vi "Main_Andor_Multi_ver2.vi"() -> ()   [LabVIEW 2014]
doc: "This is the main user interface of the Raman spectroscopy system."
uses:
  C:/Users/light/Desktop/Chuanzhen/Labview/Raman/dll/Thorlabs.MotionControl.Controls.dll
  dll/Thorlabs.MotionControl.Controls.dll
  <userlib>/atmcd64d.llb/AcquisitionMode_mode typedef.ctl
  <userlib>/atmcd64d.llb/ReadMode_mode typedef.ctl
  <userlib>/atmcd64d.llb/Shutter_mode typedef.ctl
  <userlib>/atmcd64d.llb/Shutter_type typedef.ctl
  <userlib>/atmcd64d.llb/TriggerMode_mode typedef.ctl
  TypeDef/GalvoInput.ctl
  <userlib>/atmcd64d.llb/Error Code Enum typedef.ctl
  TypeDef/States.ctl
  TypeDef/StageDeviceOut.ctl
  TypeDef/StageHandleIn.ctl
  <vilib>/Utility/miscctls.llb/LVPoint32TypeDef.ctl
  TypeDef/LaserSpot.ctl
  C:/Users/light/Desktop/Chuanzhen/Labview/Raman/dll/ThorLabs.MotionControl.KCube.DCServoCLI.dll
  dll/ThorLabs.MotionControl.KCube.DCServoCLI.dll
  TypeDef/StageSelect.ctl
  TypeDef/inputImages.ctl
  C:/Users/light/Desktop/Chuanzhen/Labview/Raman/dll/Thorlabs.MotionControl.GenericMotorCLI.dll
  dll/Thorlabs.MotionControl.GenericMotorCLI.dll
panel:
  out "Boolean":bool
  in  "Tab Control":enum32{"Main", "Andor", "Galvo"}(tab)
  in  "Scan Range":T1={"Ver_V/H"=0.35, "Hor_V/W"=0.35, "Ver_r"=5.0, "Hor_r"=5.0}
  in  "Scan Resolusion":T2={"Ver_V"=0.35, "Hor_H"=0.35, "Ver_Pix"=214.0, "Hor_Pix"=200.0}
  in  "Galvo Center":bool
  out "Galvo":bool
  out "Spot Y":dbl
  out "Spot X":dbl
  in  "Box":cluster{"Width":dbl, " Height":dbl}={"Width"=200.0, " Height"=214.0}
  in  "Quit":bool
  out "Height":i32=480
  out "Width":i32=640
  out "FPS":dbl=6.258409738085552
  in  "Blacklevel Offset":i32(slide) min=0 max=255 scale=0.0..255.0
  in  "Frame rate":dbl(slide)=9.996754624578479 min=0.5 max=17.288905497022668 step=5.487719298245614e-05 scale=0.5..17.288905497022668 scale format="%^#_3g"
  in  "Pixel clock":i32(slide)=20 min=7 max=86 scale=7.0..86.0
  in  "Exposure time (ms)":dbl(slide)=11.094175438596492 min=0.008982456140350877 max=99.9862456140351 step=0.05487719298245614 scale=0.008982456140350877..99.9862456140351 scale format="%#.3g"
  in  "Edge Filter Enable / Disable":bool
  in  "Edge Filter":i32(ring)=2 items=["High"=1, "Low"=2]
  in  "Blacklevel compensation":bool
  in  "Hotpixel correction 2":bool
  in  "Master Gain":i32(slide) min=0 max=100 scale=0.0..100.0
  in  "Autogain":bool
  out "Bits/Pixel":i32=8
  in  "Camera ID":u32
  out "Live video":picture caption="600 x 480"
  in  "Focus":bool
  out "ZoomRatio":dbl format="%#_2g"
  in  "Jog size (um)":dbl=2.0
  out "Delay (s)":dbl=0.9 format="%#_13g"
  out "Focal plane (mm)":dbl
  out "Initialization finished":bool
  in  "Aim":bool
  in  "Pixel Size X (um)":dbl=0.0877
  in  "LaserSpot":bool
  in  "Pixel Size Y (um)":dbl=0.0877
  in  "ImageSnap":bool
  in  "Left":bool
  in  "Right":bool
  in  "Up":bool
  in  "Down":bool
  in  "X axis_R":bool
  in  "X axis_L":bool
  in  "Reset":bool
  out "Z_axis":dbl
  out "X_axis":dbl
  out "Y_axis":dbl
  in  "Y axis_B":bool
  in  "Y axis_F":bool
  in  "Z axis_u":bool
  in  "Z axis_d":bool
  in  "Jogstep of Z axis":T3(radio)=enum."10step"
  in  "MoveTo":bool
  in  "Velocity: X and Y axis":T4(radio)=enum."0.05mm"
  in  "Scan":bool
  in  "Save Path":path=path "C:/Users/light/Desktop/Chuanzhen/test"
  in  "Destination":dbl=12.0
  out "Frame_X":dbl
  out "Frame_Y":dbl
  out "Total_Frame_X":dbl
  out "Total_Frame_Y":dbl
  in  "Galvo Stop":bool
  in  "Galvo Scan":bool
  out "Andor":bool
  out "CurrentFrame":i32
  in  "Set":bool
  in  "AndorSnap":bool
  out "SaveStatus":bool
  in  "FilePath":string="C:\\Users\\light\\Desktop\\Chuanzhen\\Image\\ImageReconstruct\\data\\TempSpectralData"
  in  "Exit":bool
  out "ShutDown":cluster{"CoolOff":bool, "ShutDown":bool}
  in  "Mode":T10={"AcqMode"=enum."Single Scan", "ReadMode"=enum."Single-Track", "ShutterMode"=enum."Auto", "GateMode"=enum."TTL High", "TriggerMode"=enum."Internal"}
  in  "AcqSet":T11={"openingtime"=0, "closingtime/ms"=0, "ExposureTime/s"=0.1, "AccumCycTime"=0.0, "AccumCycNum"=1, "KineticNum"=1, "KineticTime"=0.0} {"KineticTime" format="%.5f"; "AccumCycNum" format="%.5f"; "AccumCycTime" format="%.5f"; "ExposureTime/s" format="%.5f"; "closingtime/ms" format="%.2f"; "openingtime" format="%.2f"}
  out "Timing":T12 {"kinetic" format="%.7f"; "accumulate" format="%.7f"; "exposure" format="%.7f"}
  out "SetOut":T13
  in  "MultiTrack":cluster{"StartRow":i32, "EndRow":i32}={"StartRow"=131, "EndRow"=143}
  out "SetStatus":bool
  out "CurrentTemp":i32
  out "DevInit":bool
  out "DevSize":cluster{"xpixels":i32, "ypixels":i32}
  out "HardWVersion":T14
  out "SoftWVersion":T15
  out "Speeds":T16
  in  "TargetTemp":i32=-50
  out "CoolerON":T17
  out "GetStatus":T18
  in  "YOffset":dbl=8.2 caption="Offset"
  in  "XOffset":dbl=4.0 caption="Offset"
  out "Sample Rate":dbl=1000.0 format="%0.2f"
  out "Waveform Graph":waveform(dbl)[](graph)=[{"t0"=timestamp(0 s since 1904-01-01), "dt"=0.001, "Y"=[]}]
  in  "ZOffset":dbl caption="Offset"
  in  "Galvo":T19={"Sample Rate"=1000.0, "Sample Clock Source"="OnboardClock", "Max Voltage"=10.0, "Min Voltage"=-10.0, "Physical Channel(s)"="Dev1/ao0,Dev1/ao1,Dev1/ao3"}
  in  "Stage Control":enum32{"X axis", "Y axis", "Z axis"}(tab)
  in  "X axis":refnum<k24>(container)
  in  "Y axis":refnum<k24>(container)
  in  "Z axis":refnum<k24>(container)
  # "Camera Control"
  # "Objective: CFI Plan Fluor ELWD 60x (1.27 NA) \nThe depth of field: 1.78 um\nPixel Size: 0.0877um/px"
  # "Attention: \ndon't click button very fast"
  # "Motor Control"
  # "Aim"
  # "Auto Focus"
  # "Adjust laser spot lightly"
  # "Stage Scan"
  # "Total_Frame"
  # "Current_Frame"
  # "X"
  # "Y"
  # "Focus distance ia about 2mm"
  # "Jogstep:"
  # "0.00003mm/step"
  # "Stepsize:"
  # "Kinetics->SignleTrack"
  # "Galvo Control"
  # "50Hz->1s"
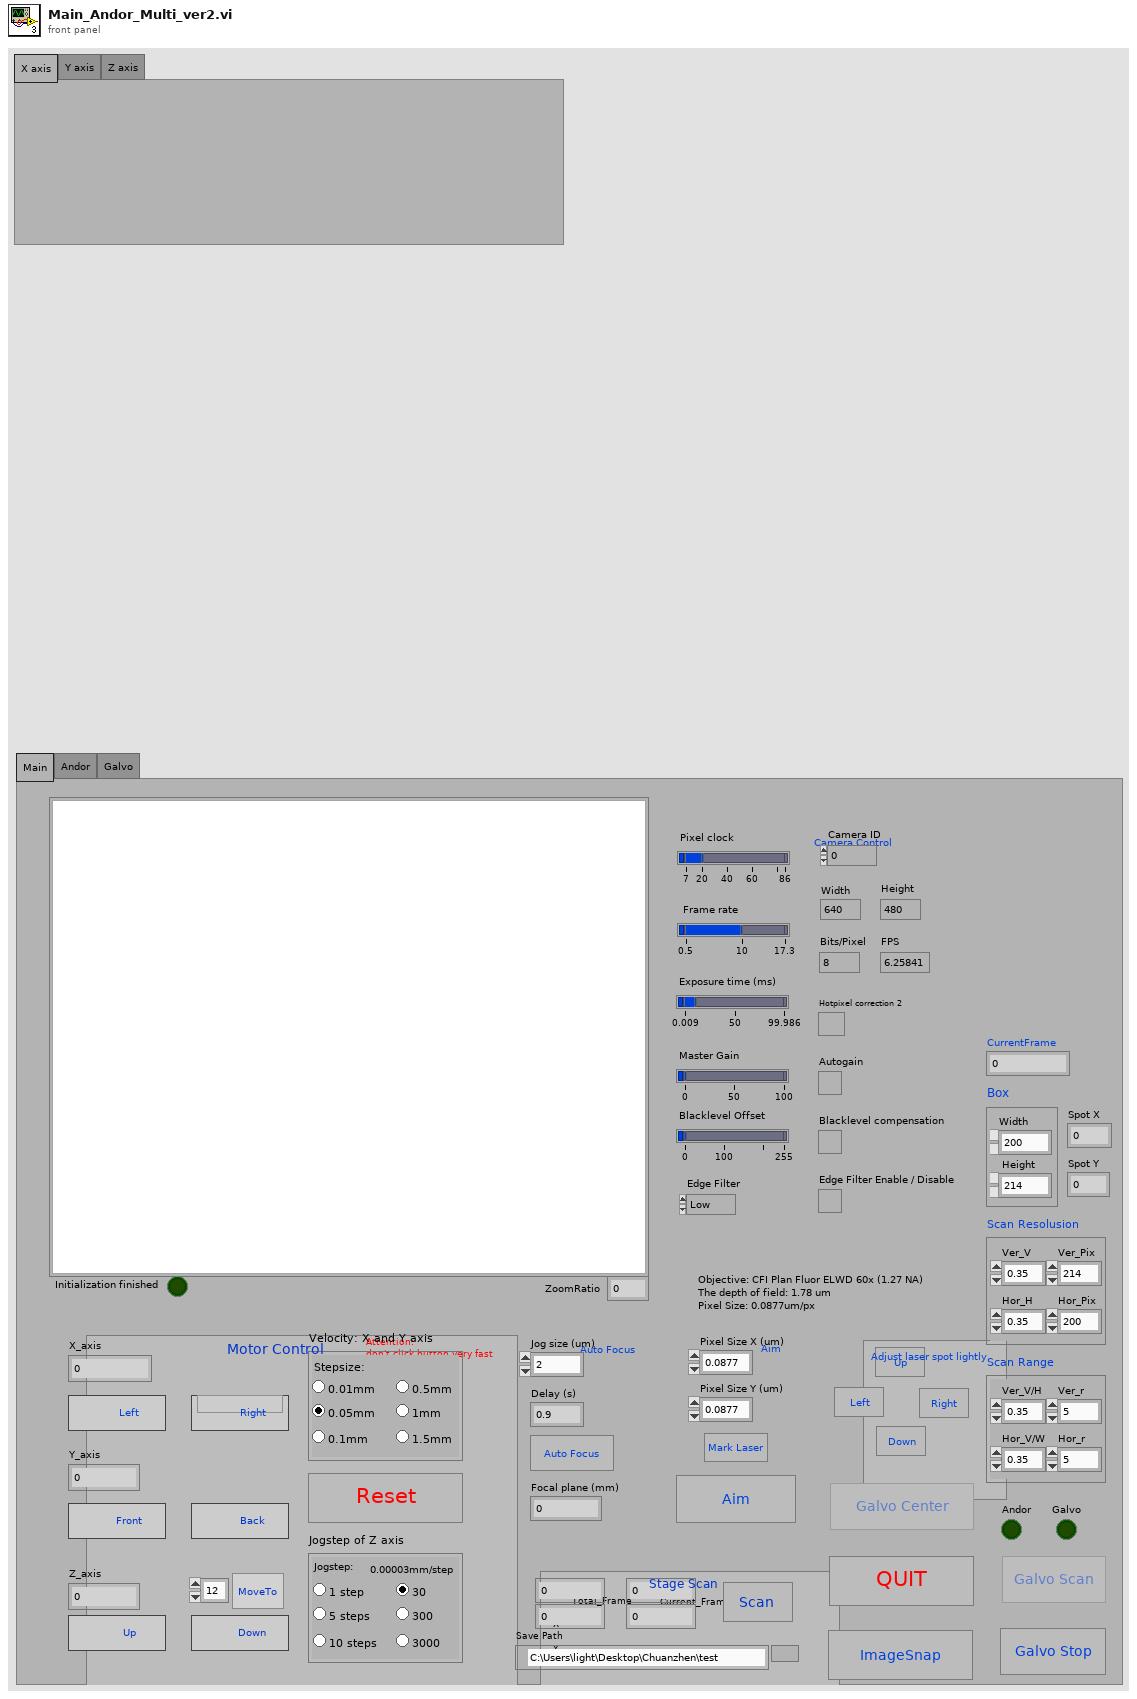
[diagram p1: front panel]
types:
  T1 = cluster{"Ver_V/H":dbl, "Hor_V/W":dbl, "Ver_r":dbl, "Hor_r":dbl}
  T2 = cluster{"Ver_V":dbl, "Hor_H":dbl, "Ver_Pix":dbl, "Hor_Pix":dbl}
  T3 = enum32{"1step", "2step", "5step", "10step", "15step", "20step"}
  T4 = enum32{"0.01mm", "0.05mm", "0.1mm", "0.5mm", "1mm", "1.5mm"}
  T5 = typedef "AcquisitionMode_mode typedef.ctl" = enum16{"Reserved (0)", "Single Scan", "Accumulate", "Kinetics", "Fast Kinetics", "Run Till Abort", "Reserved (6)", "Reserved (7)", "Reserved (8)", "Time Delayed Integration"}
  T6 = typedef "ReadMode_mode typedef.ctl" = enum16{"Full Vertical Binning", "Multi-Track", "Random-Track", "Single-Track", "Image"}
  T7 = typedef "Shutter_mode typedef.ctl" = enum16{"Auto", "Open", "Close", "N/A (3)", "Open FVB Series", "Open Any Series"}
  T8 = typedef "Shutter_type typedef.ctl" = enum16{"TTL Low", "TTL High"}
  T9 = typedef "TriggerMode_mode typedef.ctl" = enum16{"Internal", "External", "N/A (2)", "N/A (3)", "N/A (4)", "N/A (5)", "External Start", "External Exposure (Bulb)", "N/A (8)", "External FVB EM", "Software", "N/A (11)", "External Charge Shifting"}
  T10 = cluster{"AcqMode":T5, "ReadMode":T6, "ShutterMode":T7, "GateMode":T8, "TriggerMode":T9}
  T11 = cluster{"openingtime":i32, "closingtime/ms":i32, "ExposureTime/s":sgl, "AccumCycTime":sgl, "AccumCycNum":i32, "KineticNum":i32, "KineticTime":sgl}
  T12 = cluster{"exposure":sgl, "accumulate":sgl, "kinetic":sgl}
  T13 = cluster{"Height":i32, "Width":i32, "bottom":i32, "gap":i32}
  T14 = cluster{"PCB":u32, "Flex":u32, "dummy1":u32, "dummy2":u32, "dummy3":u32, "dummy4":u32}
  T15 = cluster{"eprom":u32, "cofFile":u32, "vxdRev":u32, "vxdVer":u32, "dllRev":u32, "dllVer":u32}
  T16 = cluster{"NVS":i32, "VS":i32, "NHS":dbl, "HS":i32}
  T17 = cluster{"SetTemp":bool, "CoolerOn":bool, "Stablized":bool}
  T18 = cluster{"GetDetector":bool, "GetHardVer":bool, "GetNVS":bool, "GetVS":bool, "GetSotfVer":bool, "GetNHS":bool, "GetHS":bool}
  T19 = typedef "GalvoInput.ctl" = cluster{"Sample Rate":dbl, "Sample Clock Source":tag, "Max Voltage":dbl, "Min Voltage":dbl, "Physical Channel(s)":tag}
  T20 = typedef "LaserSpot.ctl" = cluster{"Laser X":dbl, "Laser Y":dbl}
  T21 = cluster{"left":i16, "top":i16, "right":i16, "bottom":i16}
  T22 = typedef "LVPoint32TypeDef.ctl" = cluster{"Horizontal":i32, "Vertical":i32}
  T23 = typedef "StageHandleIn.ctl" = cluster{"Z StageHandle in":refnum<k24>, "X StageHandle in":refnum<k24>, "Y StageHandle in":refnum<k24>}
  T24 = typedef "StageDeviceOut.ctl" = cluster{"Device Z":refnum<k24>, "Device X":refnum<k24>, "Device Y":refnum<k24>}
  T25 = typedef "States.ctl" = enum16{"Initialize", "CMOS live", "Shut down"}
  T26 = enum8{"Enabled", "Disabled", "Disabled and Grayed Out"}
  T27 = cluster{"Width":u16, "Style":enum32{"Solid", "Dash", "Dot", "DashDot", "DashDotDot"}}
  T28 = typedef "StageSelect.ctl" = enum16{"X axis", "Y axis", "Z axis"}
  T29 = typedef "inputImages.ctl" = cluster{"Image2":u8[][], "Image3":u8[][], "Image4":u8[][], "Image1":u8[][]}
  T30 = typedef "Error Code Enum typedef.ctl" = enum32{"N/A (0)", "DRV_ERROR_CODES", "DRV_SUCCESS", "DRV_VXDNOTINSTALLED", "DRV_ERROR_SCAN", "DRV_ERROR_CHECK_SUM", "DRV_ERROR_FILELOAD", "DRV_UNKNOWN_FUNC", "DRV_ERROR_VXD_INIT", "DRV_ERROR_ADDRESS", "DRV_ERROR_PAGELOCK", "DRV_ERROR_PAGEUNLOCK", "DRV_ERROR_BOARDTEST", "DRV_ERROR_ACK", "DRV_ERROR_UP_FIFO", "DRV_ERROR_PATTERN", "N/A (16)", "DRV_ACQUISITION_ERRORS", "DRV_ACQ_BUFFER", "DRV_ACQ_DOWNFIFO_FULL", "DRV_PROC_UNKONWN_INSTRUCTION", "DRV_ILLEGAL_OP_CODE", "DRV_KINETIC_TIME_NOT_MET", "DRV_ACCUM_TIME_NOT_MET", "DRV_NO_NEW_DATA", "N/A (25)", "DRV_SPOOLERROR", "N/A (27)", "N/A (28)", "N/A (29)", "N/A (30)", "N/A (31)", "N/A (32)", "DRV_TEMPERATURE_CODES", "DRV_TEMPERATURE_OFF", "DRV_TEMPERATURE_NOT_STABILIZED", "DRV_TEMPERATURE_STABILIZED", "DRV_TEMPERATURE_NOT_REACHED", "DRV_TEMPERATURE_OUT_RANGE", "DRV_TEMPERATURE_NOT_SUPPORTED", "DRV_TEMPERATURE_DRIFT", "N/A (41)", "N/A (42)", "N/A (43)", "N/A (44)", "N/A (45)", "N/A (46)", "N/A (47)", "N/A (48)", "DRV_GENERAL_ERRORS", "DRV_INVALID_AUX", "DRV_COF_NOTLOADED", "DRV_FPGAPROG", "DRV_FLEXERROR", "DRV_GPIBERROR", "N/A (55)", "N/A (56)", "N/A (57)", "N/A (58)", "N/A (59)", "N/A (60)", "N/A (61)", "N/A (62)", "N/A (63)", "DRV_DATATYPE", "DRV_DRIVER_ERRORS", "DRV_P1INVALID", "DRV_P2INVALID", "DRV_P3INVALID", "DRV_P4INVALID", "DRV_INIERROR", "DRV_COFERROR", "DRV_ACQUIRING", "DRV_IDLE", "DRV_TEMPCYCLE", "DRV_NOT_INITIALIZED", "DRV_P5INVALID", "DRV_P6INVALID", "DRV_INVALID_MODE", "DRV_INVALID_FILTER", "DRV_I2CERRORS", "DRV_I2CDEVNOTFOUND", "DRV_I2CTIMEOUT", "DRV_P7INVALID", "N/A (84)", "N/A (85)", "N/A (86)", "N/A (87)", "N/A (88)", "N/A (89)", "DRV_IOCERROR", "DRV_VRMVERSIONERROR"}
  T31 = typedef "StageHandleOut.ctl" = cluster{"Z StageHandle out":refnum<k24>, "X StageHandle out":refnum<k24>, "Y StageHandle out":refnum<k24>}
  T32 = typedef "LVBoundsTypeDef.ctl" = cluster{"Width":u32, "Height":u32}
  T33 = typedef "imagedata.ctl" = cluster{"image type":i32, "image depth":i32, "image":u8[], "mask":u8[], "colors":u32[], "Rectangle":cluster{"left":i16, "top":i16, "right":i16, "bottom":i16}}
  T34 = typedef "LVPositionTypeDef.ctl" = cluster{"Left":i32, "Top":i32}
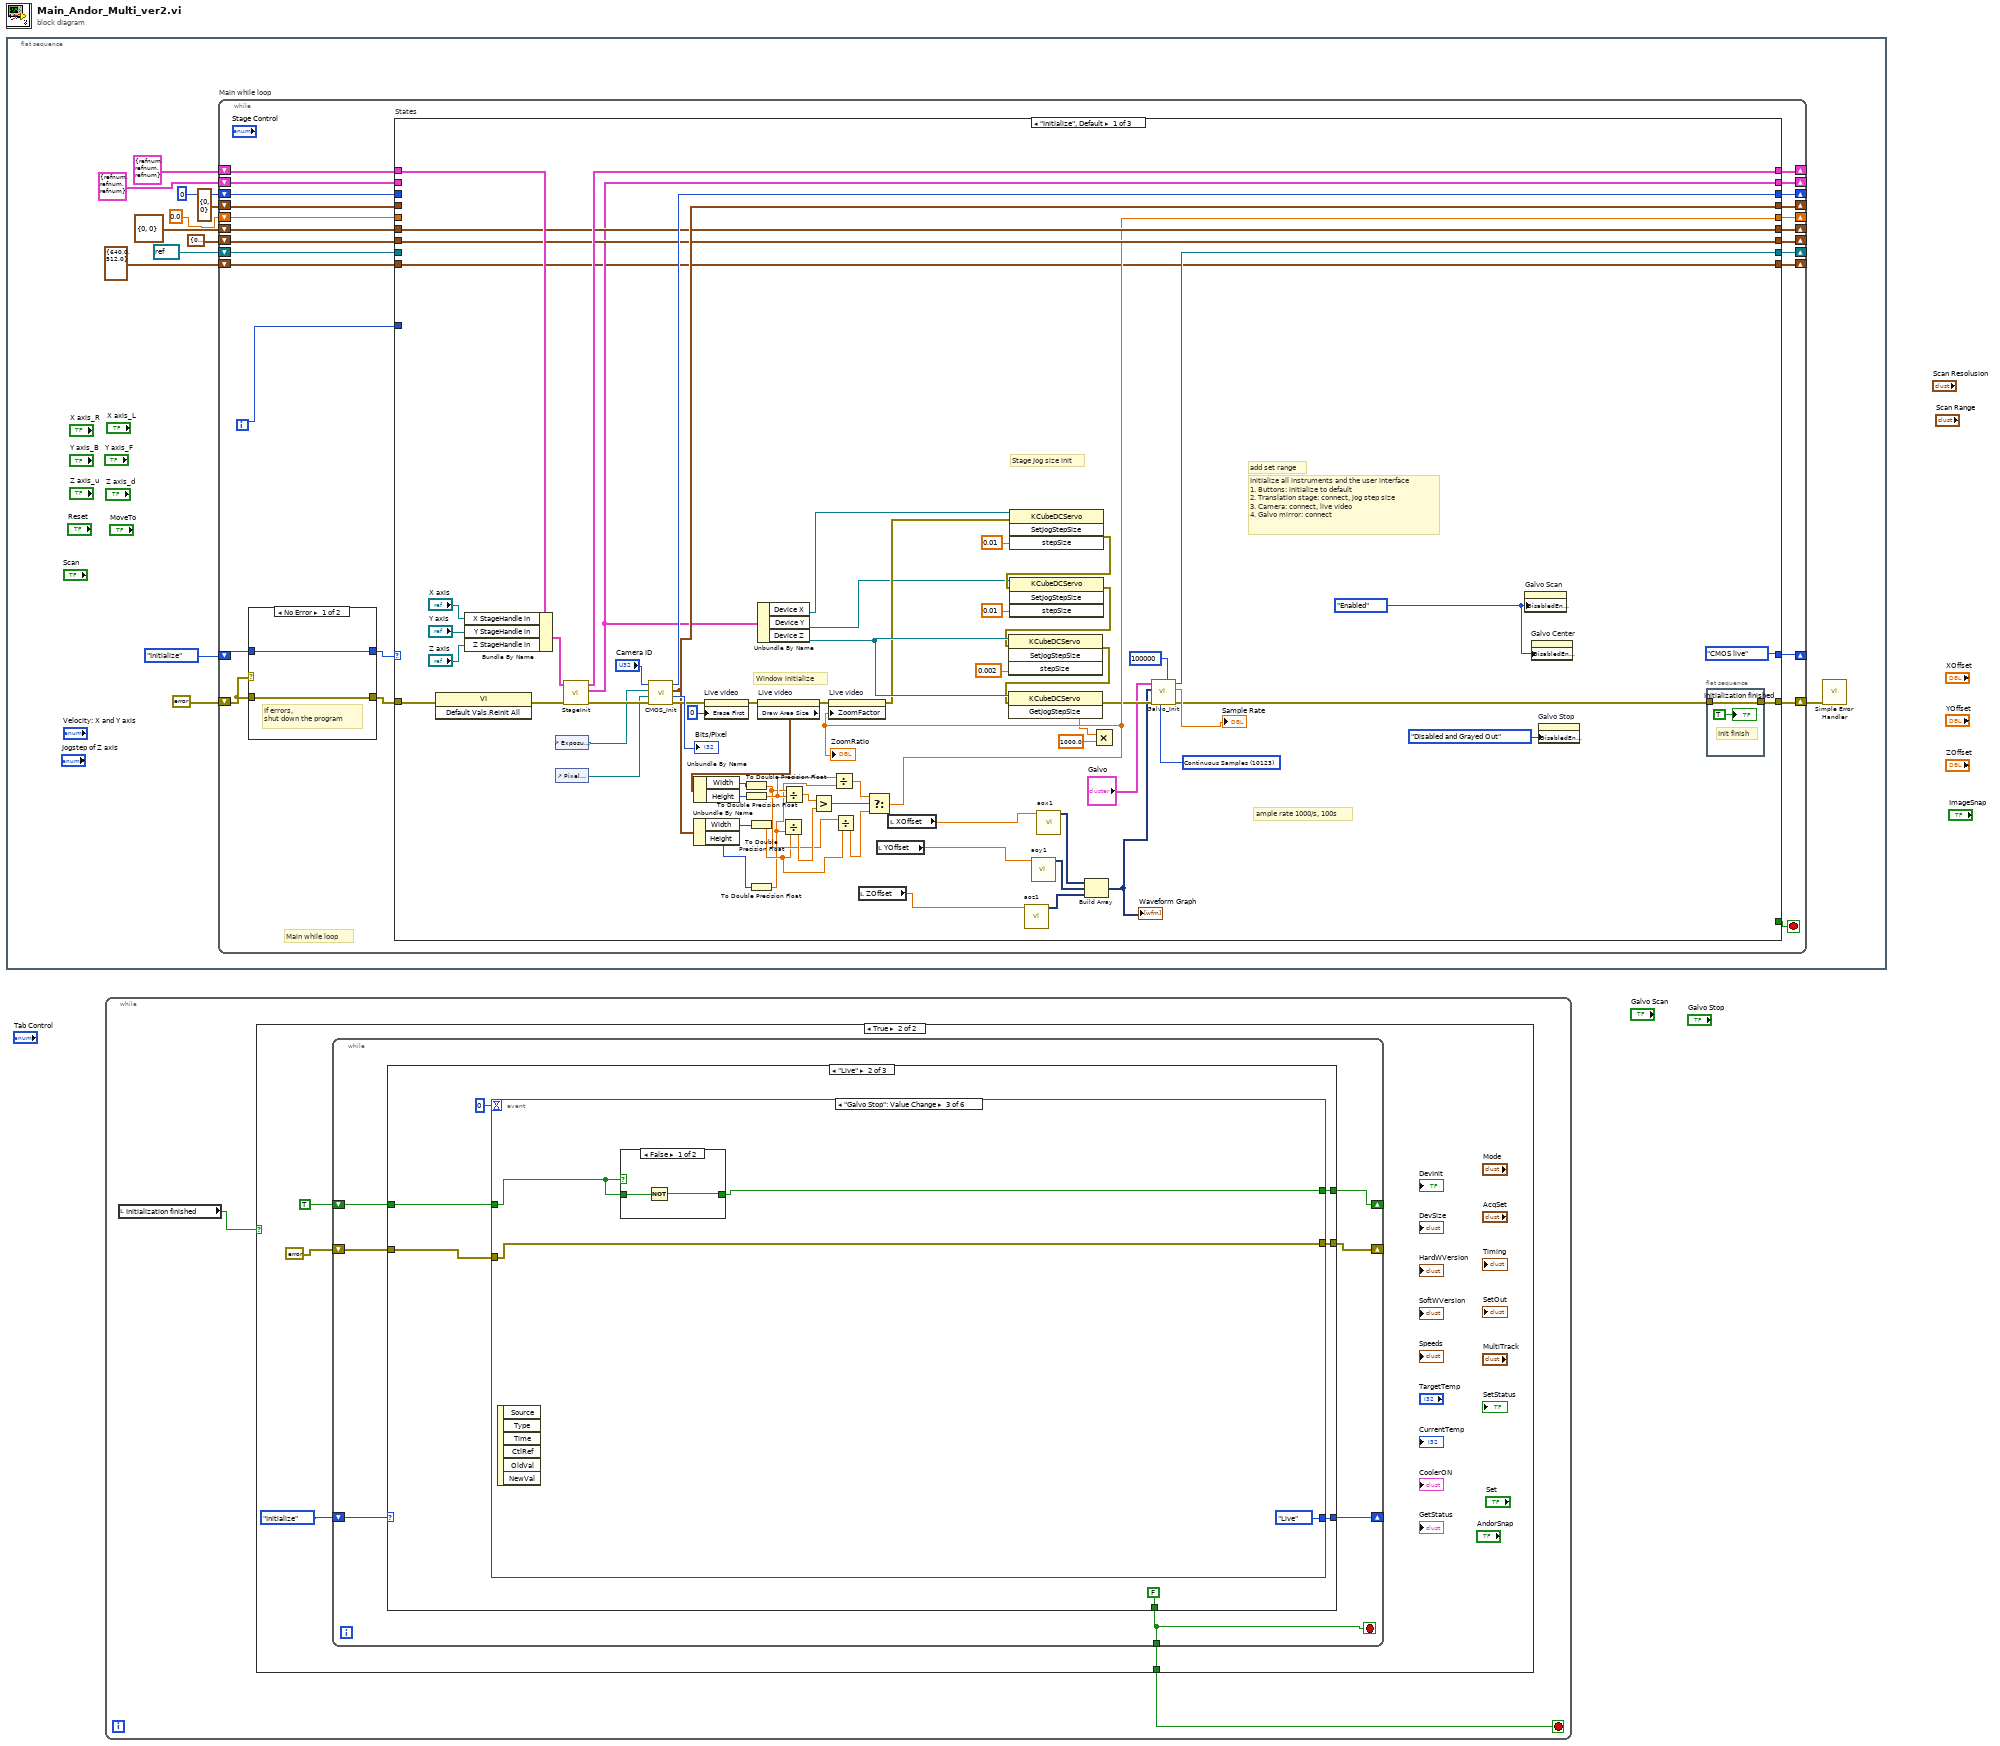
[diagram p0: block diagram]
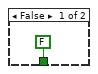
[diagram p2: hidden frame]
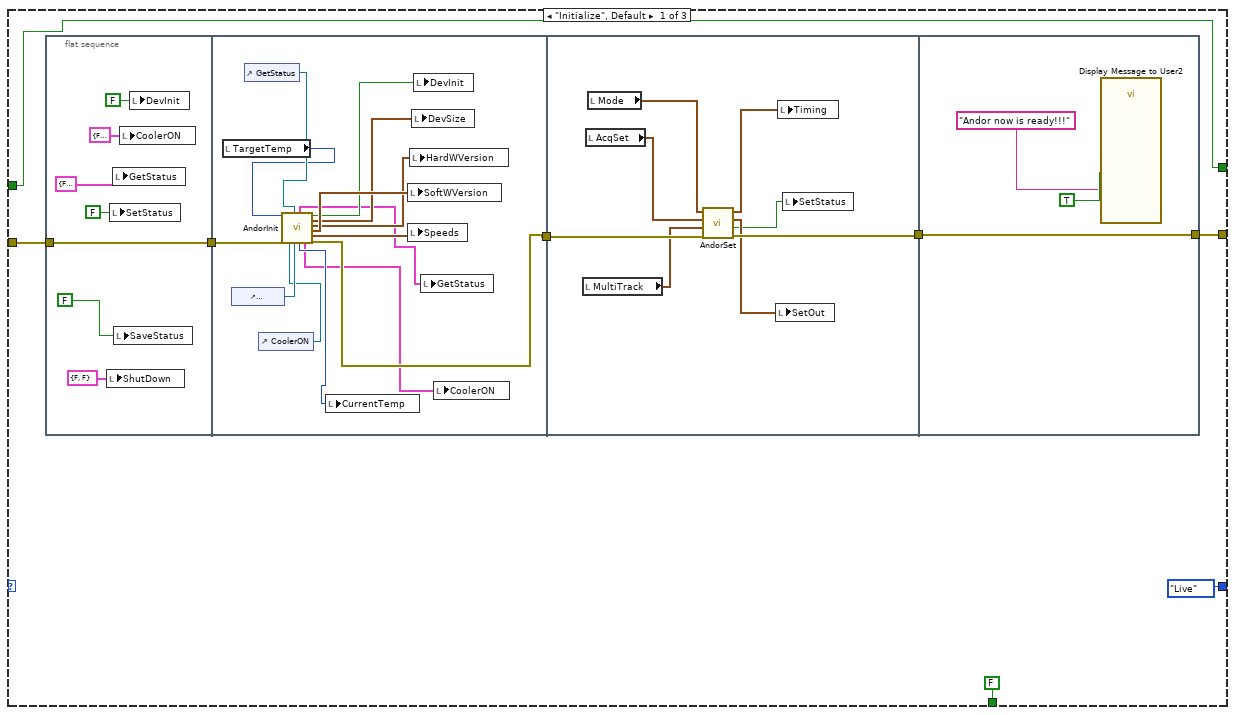
[diagram p3: hidden frame]
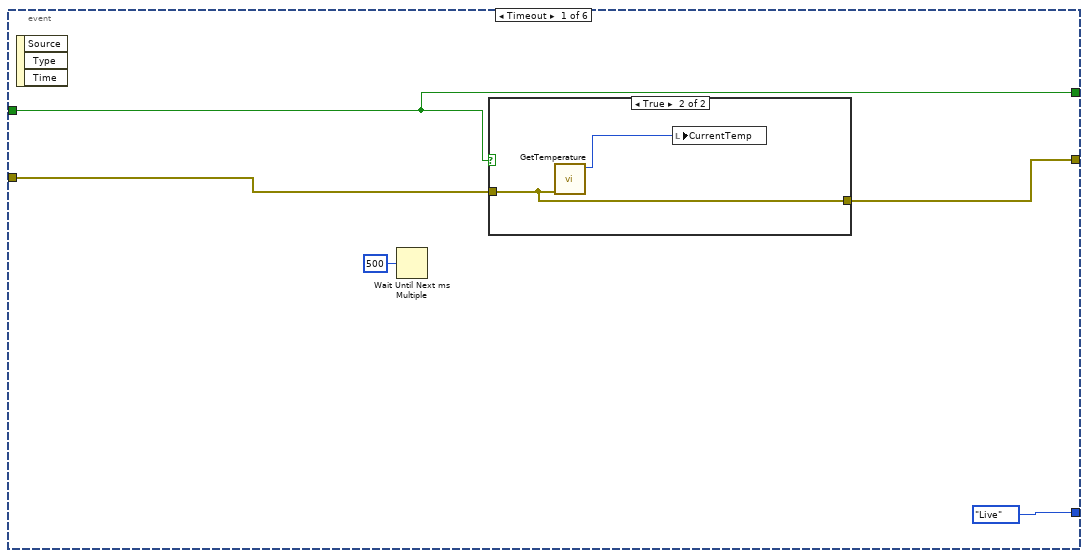
[diagram p4: hidden frame]
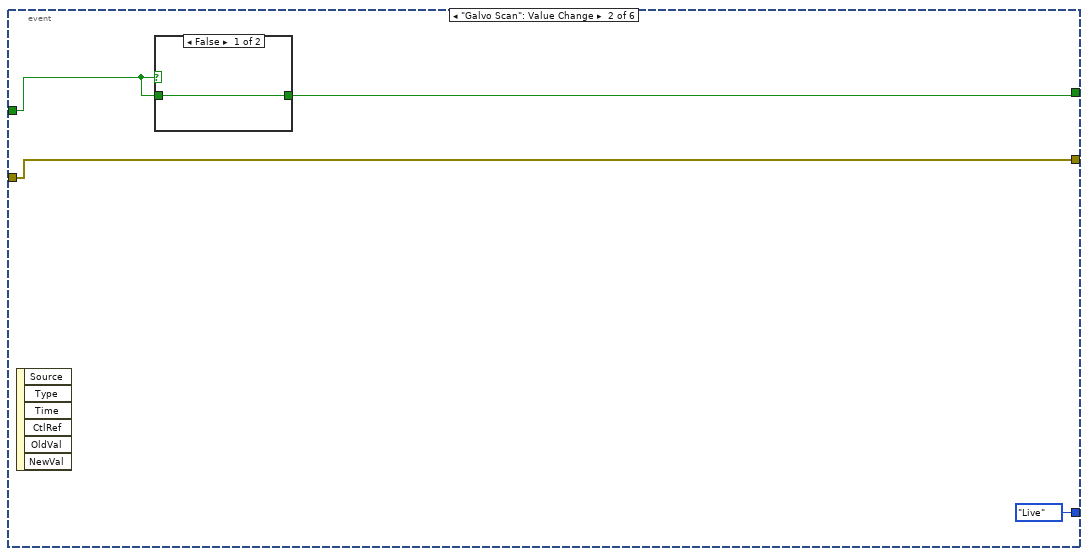
[diagram p6: hidden frame]
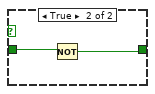
[diagram p7: hidden frame]
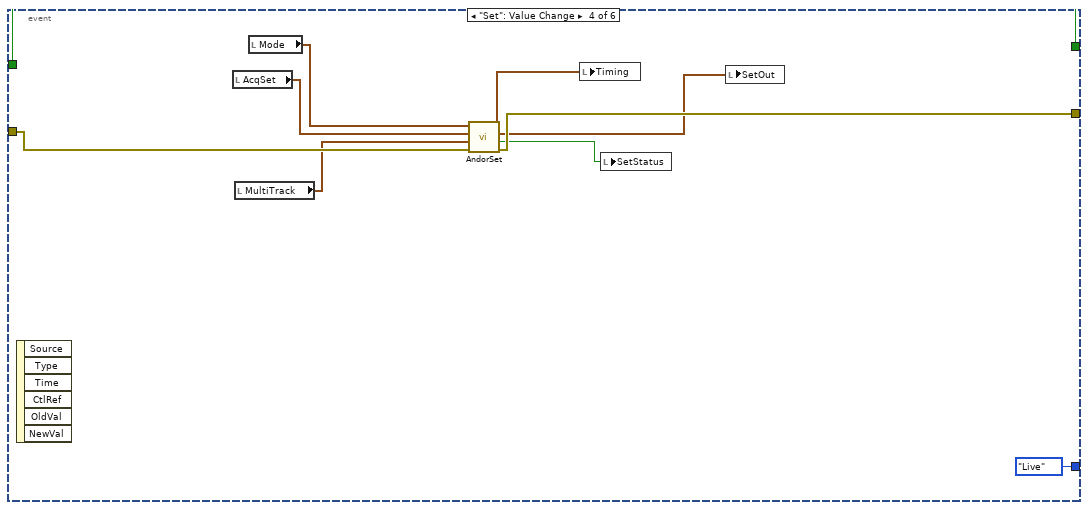
[diagram p9: hidden frame]
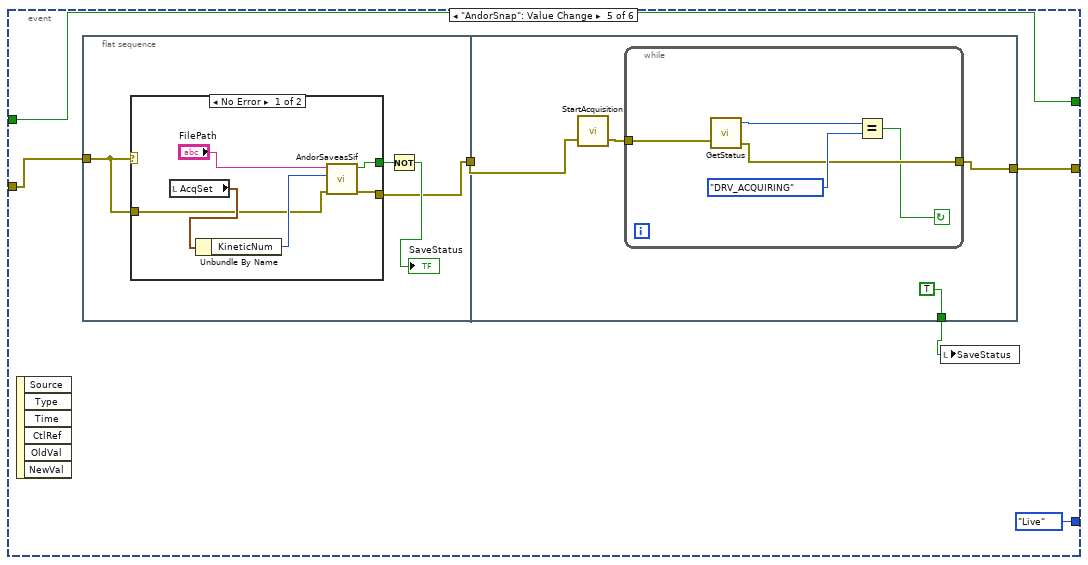
[diagram p10: hidden frame]
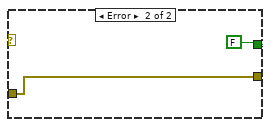
[diagram p11: hidden frame]
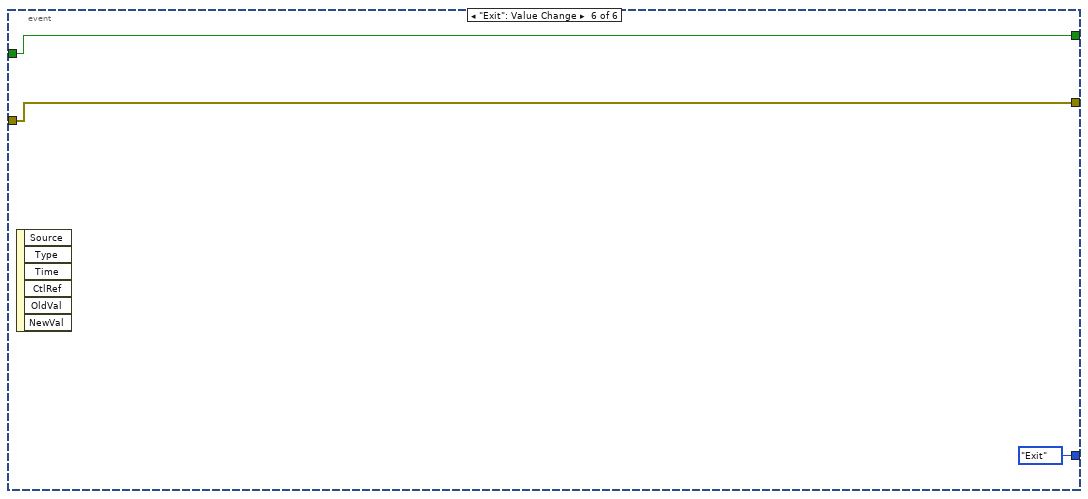
[diagram p12: hidden frame]
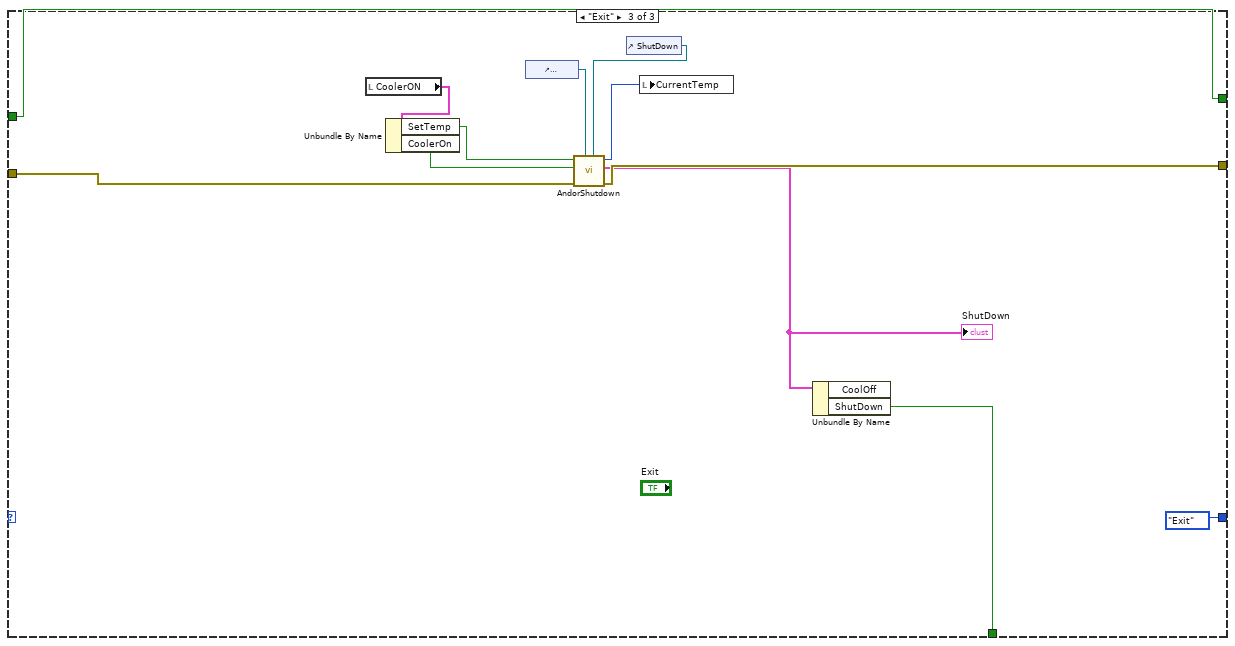
[diagram p13: hidden frame]
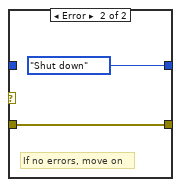
[diagram p14: hidden frame]
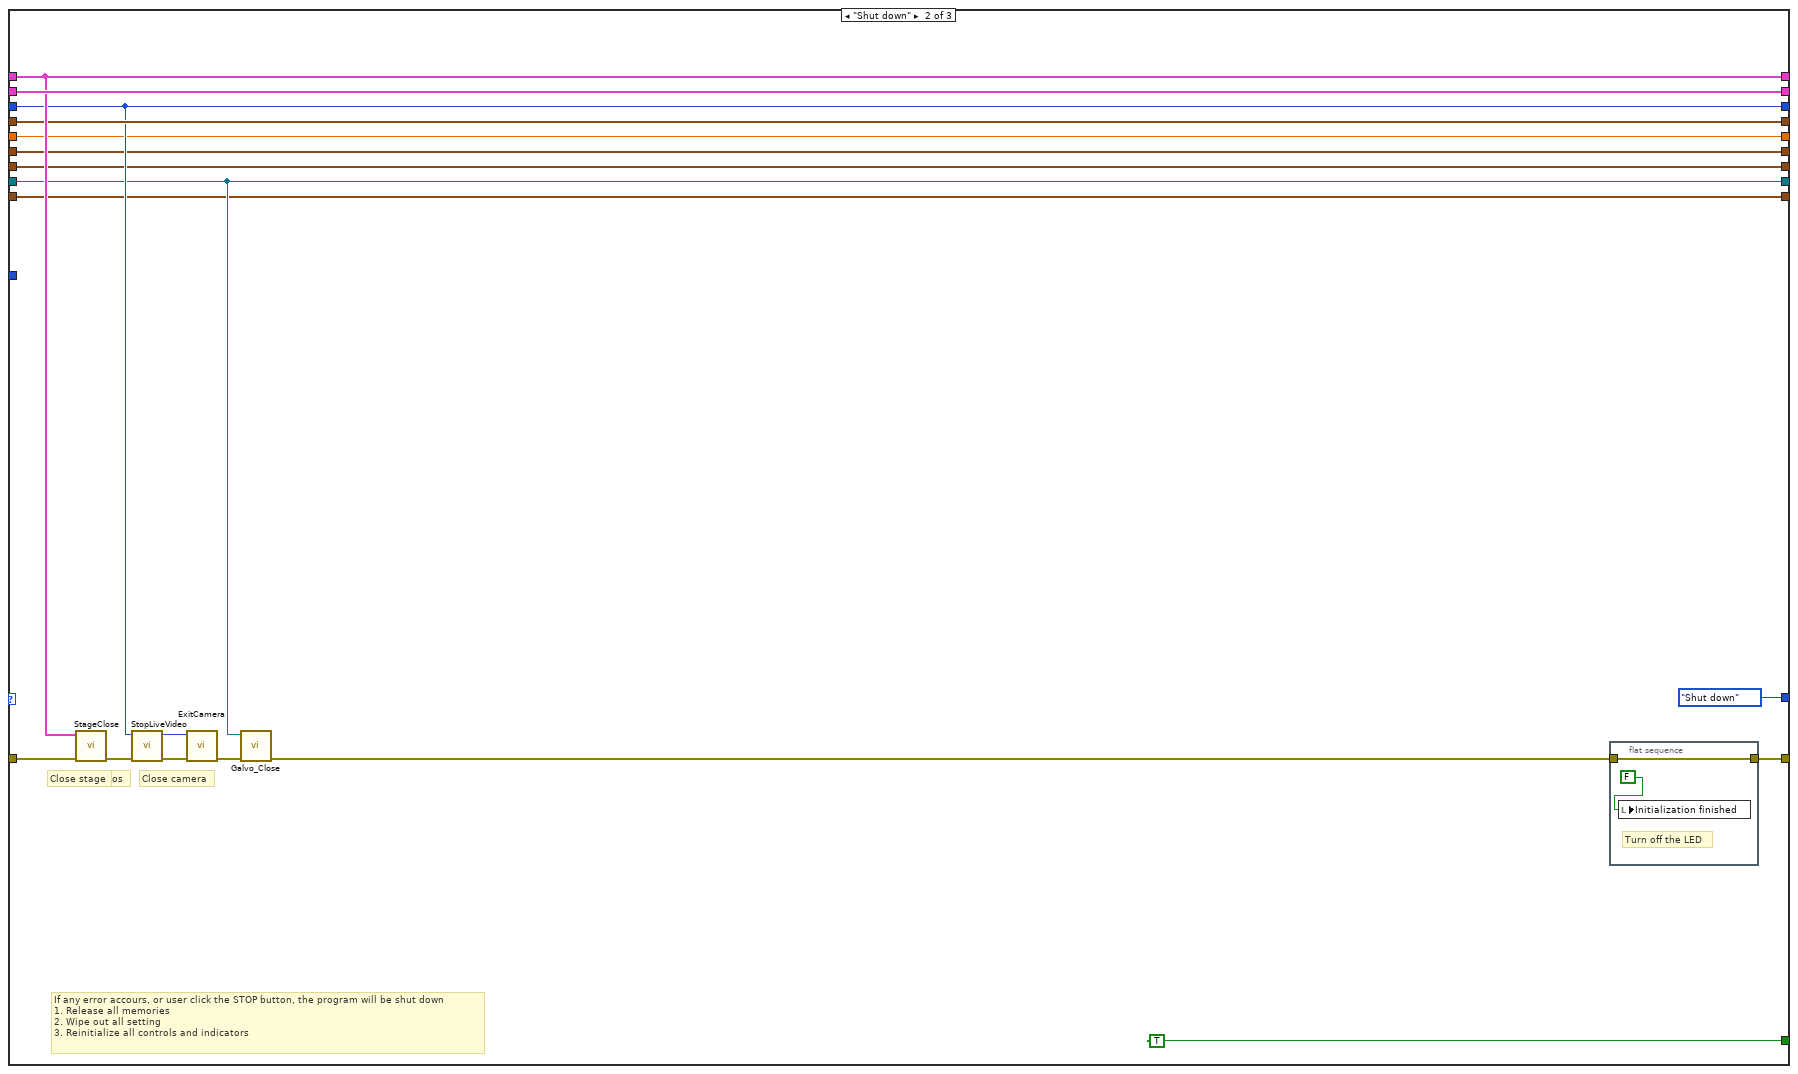
[diagram p15: hidden frame]
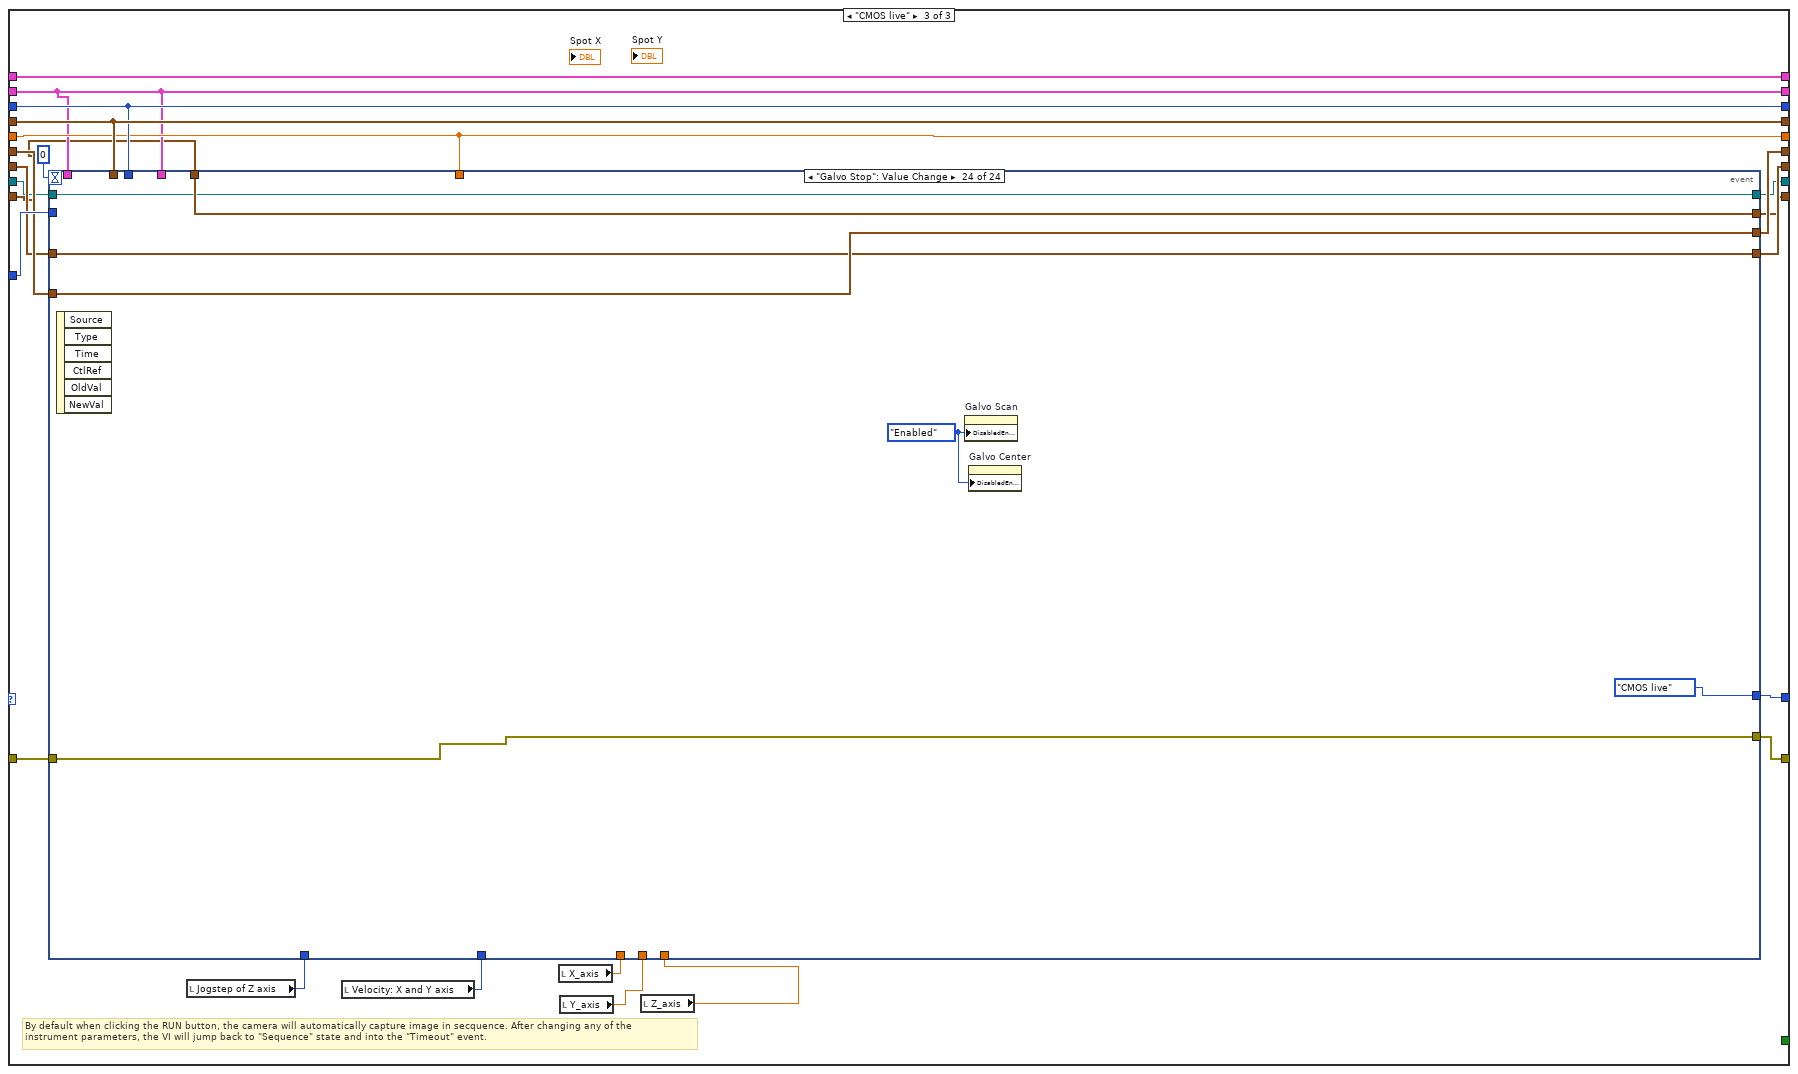
[diagram p16: hidden frame]
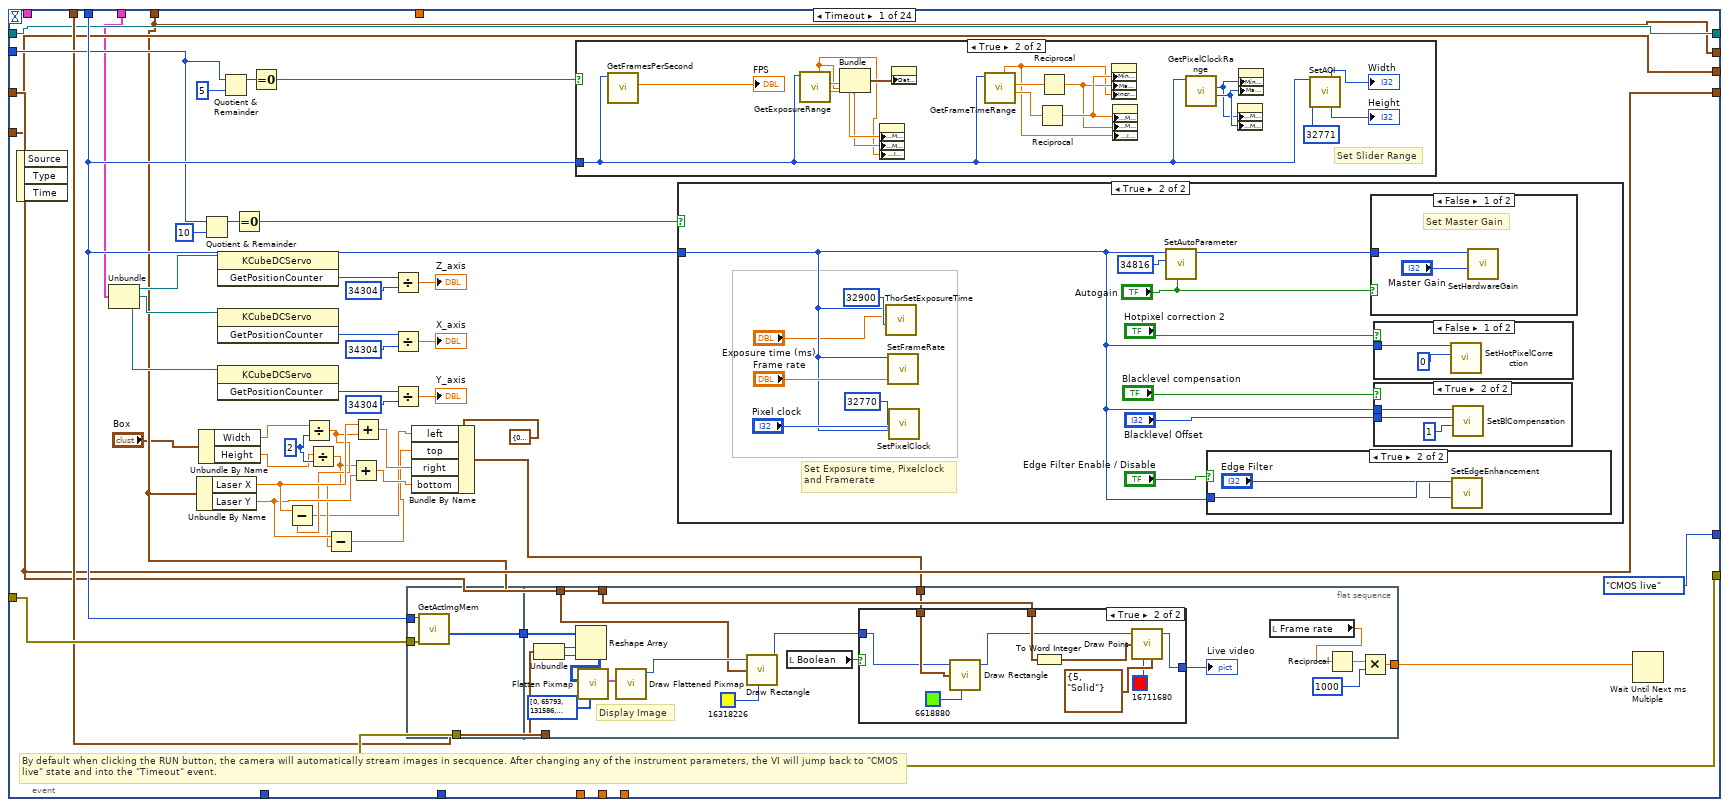
[diagram p17: hidden frame]
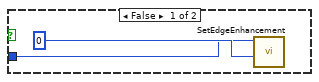
[diagram p19: hidden frame]
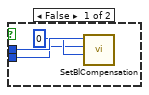
[diagram p20: hidden frame]
diagram:
  n1 = flat-sequence {
    frame #0 {
      n2 = while "Main while loop" {
        shift-right: [w33] -> _
        shift-left: States."Initialize" -> [w38]
        shift-right: [w36] -> w10
        shift-left: errorcluster {"status"=FALSE, "code"=0, "source"=""} ("error out") -> [w32]
        shift-right: [w30] -> _
        shift-left: T23 {"Z StageHandle in"=refnum, "X StageHandle in"=refnum, "Y StageHandle in"=refnum} ("StageHandle In") -> [w31]
        shift-right: [w29] -> _
        shift-left: T24 {"Device Z"=refnum, "Device X"=refnum, "Device Y"=refnum} ("Device Out") -> [w28]
        shift-right: [w27] -> _
        shift-left: u32 0 ("CMOS Handle Out") -> [w26]
        shift-right: [w24] -> _
        shift-left: cluster{"Height":i32, "Width":i32} {"Height"=0, "Width"=0} ("WidthAndHeight") -> [w23]
        shift-right: [w22] -> _
        shift-left: 0.0 -> [w17]
        shift-right: [w21] -> _
        shift-left: T22 {"Horizontal"=0, "Vertical"=0} ("Coords") -> [w20]
        shift-right: [w19] -> _
        shift-left: T21 {"left"=0, "top"=0, "right"=0, "bottom"=0} ("rect") -> [w18]
        shift-right: [w16] -> _
        shift-left: refnum<k21> refnum ("task out") -> [w15]
        shift-right: [w14] -> _
        shift-left: T20 {"Laser X"=640.0, "Laser Y"=512.0} ("LaserSpot 2") -> [w13]
        i -> [w25]
        stop <- w34 stop-if-true
        # "Main while loop"
        n3 = case shown="No Error" w32 {
          tunnel: w32 -> [w40 w42]
          tunnel: [w40 w42] -> w35
          tunnel: w38 -> [w39 _]
          tunnel: [w39 States."Shut down"] -> w37
          frame No Error {
            # "If errors,\nshut down the program"
          }
          frame Error {
            # "If no errors, move on"
          }
        }
        n4 = case "States" shown="\"Initialize\", Default" w37 {
          tunnel: [w68 w117 w152] -> w36
          tunnel: w35 -> [w109 w127 w153]
          tunnel: [_ TRUE _] -> w34
          tunnel: [States."CMOS live" States."Shut down" w154] -> w33
          tunnel: w31 -> [w107 w126 w155]
          tunnel: [w106 w126 w155] -> w30
          tunnel: [w73 w128 w142] -> w29
          tunnel: w28 -> [_ w128 w142]
          tunnel: [w100 w121 w148] -> w27
          tunnel: w26 -> [_ w121 w148]
          tunnel: w25 -> [_ _ w150]
          tunnel: [w81 w125 w149] -> w24
          tunnel: w23 -> [_ w125 w149]
          tunnel: [w74 w120 w143] -> w22
          tunnel: w17 -> [_ w120 w143]
          tunnel: [w76 w119 w147] -> w21
          tunnel: w20 -> [w76 w119 w146]
          tunnel: [w75 w118 w145] -> w19
          tunnel: w18 -> [w75 w118 w144]
          tunnel: [w56 w115 w140] -> w16
          tunnel: w15 -> [_ w115 w141]
          tunnel: [w52 w113 w139] -> w14
          tunnel: w13 -> [w52 w113 w138]
          frame "Initialize", Default {
            w44 = T26."Enabled" ("Disabled")
            w50 = 10123 items=["Finite Samples"=10178, "Continuous Samples"=10123, "Hardware Timed Single Point"=12522] ("Sample Mode")
            # "ample rate 1000/s, 100s"
            # "add set range"
            # "Stage Jog size init"
            # "Window initialize"
            # "Initialize all instruments and the user interface\n1. Buttons: initialize to default\n2. Translation stage: connect, jog step size\n3. Camera: connect, live video\n4. Galvo mirror: connect"
            n5 = invoke class="VI" method="Default Vals.Reinit All"(error in=w109) -> (error out=w108:errorcluster)  [unwired: 2 in, 2 out]
            n6 = Bundle By Name(cluster=w107, "X StageHandle in"="X axis", "Y StageHandle in"="Y axis", "Z StageHandle in"="Z axis") -> (w105:T23)
            n7 = control-ref of="Exposure time (ms)"() -> (w99:refnum<vi>)
            n8 = control-ref of="Pixel clock"() -> (w98:refnum<vi>)
            n9 = call "StageInit.vi"("error in (no error)"=w108, "StageHandle In"=w105) -> ("error out"=w101:errorcluster, "Device Out"=w73:T24, "StageHandle Out"=w106:T31)  [unwired: 7 in]
            n10 = call "CMOS_Init.vi"("error in"=w101, "Pixel clock"=w98, "Exposure time"=w99, "Camera ID"="Camera ID") -> ("error out"=w95:errorcluster, "Bits/Pixel"=→"Bits/Pixel":i32, "WidthAndHeight"=w81:cluster{"Height":i32, "Width":i32}, "CMOS Handle Out"=w100:u32)  [unwired: 3 in]
            n11 = Unbundle By Name(w81) -> ("Width"=w80:i32, "Height"=w79:i32)
            n12 = property on="Live video" class="Pict"(error in=w95, "Erase First"=u8 0) -> (error out=w83:errorcluster)  [unwired: 1 in, 1 out]
            n13 = To Double Precision Float(number=w80) -> (double precision float=w78:dbl)
            n14 = To Double Precision Float(number=w79) -> (double precision float=w77:dbl)
            n15 = Unbundle By Name(w73) -> ("Device X"=w61:refnum<k24>, "Device Y"=w60:refnum<k24>, "Device Z"=w71:refnum<k24>)
            n16 = property on="Live video" class="Pict"(error in=w83) -> (error out=w82:errorcluster, "Draw Area Size"=w93:T32)  [unwired: 1 in, 1 out]
            n17 = Unbundle By Name(w93) -> ("Width"=w91:u32, "Height"=w92:u32)
            n18 = To Double Precision Float(number=w91) -> (double precision float=w85:dbl)
            n19 = To Double Precision Float(number=w92) -> (double precision float=w87:dbl)
            n20 = Divide(x=w78, y=w77) -> (x/y=w88:dbl)
            n21 = Divide(x=w85, y=w87) -> (x/y=w90:dbl)
            n22 = Greater?(x=w90, y=w88) -> (0:w89:bool)
            n23 = Divide(x=w87, y=w77) -> (x/y=w86:dbl)
            n24 = Divide(x=w85, y=w78) -> (x/y=w84:dbl)
            n25 = local read "ZOffset"() -> (w45:dbl)
            n26 = Select(t=w86, s=w89, f=w84) -> (s? t:f=w74:dbl)
            "ZoomRatio" <- w74
            n27 = property on="Live video" class="Pict"(error in=w82, "ZoomFactor"=w74) -> (error out=w64:errorcluster)  [unwired: 1 in, 1 out]
            n28 = local read "YOffset"() -> (w46:dbl)
            n29 = local read "XOffset"() -> (w47:dbl)
            n30 = invoke class="KCubeDCServo" method="SetJogStepSize"(reference=w61, error in=w64, "stepSize"=0.01) -> (error out=w63:errorcluster)  [unwired: 1 in, 3 out]
            n31 = invoke class="KCubeDCServo" method="SetJogStepSize"(reference=w60, error in=w63, "stepSize"=0.01) -> (error out=w62:errorcluster)  [unwired: 1 in, 3 out]
            n32 = invoke class="KCubeDCServo" method="SetJogStepSize"(reference=w71, error in=w62, "stepSize"=0.002) -> (error out=w70:errorcluster)  [unwired: 1 in, 3 out]
            n33 = invoke class="KCubeDCServo" method="GetJogStepSize"(reference=w71, error in=w70) -> (error out=w59:errorcluster, "GetJogStepSize"=w69:dbl)  [unwired: 1 in, 1 out]
            n34 = call "aoz1"("Offset"=w45) -> ("DC"=w54:dynamicdata)  [unwired: 13 in, 1 out]
            n35 = call "aoy1"("Offset"=w46) -> ("DC"=w48:dynamicdata)  [unwired: 13 in, 1 out]
            n36 = call "aox1"("Offset"=w47) -> ("DC"=w49:dynamicdata)  [unwired: 13 in, 1 out]
            n37 = Build Array(w49, w48, w54) -> (w53:dynamicdata[])
            "Waveform Graph" <- w53
            n38 = Multiply(x=w69, y=1000.0) -> ()  [unwired: 1 out]
            n39 = call "Galvo_Init.vi"("Sample Mode"=w50, "samples per channel"=100000, "error in"=w59, "Signal array"=w53, "Galvo_Input"="Galvo") -> ("error out"=w55:errorcluster, "Actual Sample Rate"=→"Sample Rate":dbl, "task out"=w56:refnum<k21>)  [unwired: 4 in]
            n40 = property on="Galvo Scan" class="Bool"("DisabledEnum"=w44) -> ()  [unwired: 2 in, 2 out]
            n41 = property on="Galvo Center" class="Bool"("DisabledEnum"=w44) -> ()  [unwired: 2 in, 2 out]
            n42 = property on="Galvo Stop" class="Bool"("DisabledEnum"=T26."Disabled and Grayed Out" ("Disabled")) -> ()  [unwired: 2 in, 2 out]
            n43 = flat-sequence {
              tunnel: w55 -> [w112]
              tunnel: [w112] -> w68
              frame #0 {
                # "Init finish"
                "Initialization finished" <- TRUE ("Initialization finished")
              }
            }
          }
          frame "Shut down" {
            # "Close 3 galvos"
            # "Close camera"
            # "Close stage"
            # "If any error accours, or user click the STOP button, the program will be shut down\n1. Release all memories\n2. Wipe out all setting\n3. Reinitialize all controls and indicators"
            n44 = call "StageClose.vi"("error in (no error)"=w127, "StageHandle In"=w126) -> ("error out"=w124:errorcluster)  [unwired: 9 in]
            n45 = call "StopLiveVideo.vi"("error in"=w124, "Camera Handle In"=w121) -> ("error out"=w123:errorcluster, "Camera Handle Out"=w122:u32)  [unwired: 8 in]
            n46 = call "ExitCamera.vi"("error in"=w123, "Camera Handle In"=w122) -> ("error out"=w116:errorcluster)  [unwired: 9 in]
            n47 = call "Galvo_Close.vi"("error in"=w116, "task/channels in"=w115) -> ("error out"=w114:errorcluster)  [unwired: 9 in]
            n48 = flat-sequence {
              tunnel: w114 -> [w132]
              tunnel: [w132] -> w117
              frame #0 {
                # "Turn off the LED"
                n49 = local write "Initialization finished"(FALSE ("Initialization finished")) -> ()
              }
            }
          }
          frame "CMOS live" {
            # "By default when clicking the RUN button, the camera will automatically capture image in secquence. After changing any of the \ninstrument parameters, the VI will jump back to \"Sequence\" state and into the \"Timeout\" event."
            n50 = local read "Jogstep of Z axis"() -> (w133:T3)
            n51 = local read "Velocity: X and Y axis"() -> (w137:T4)
            n52 = local read "X_axis"() -> (w136:dbl)
            n53 = local read "Y_axis"() -> (w135:dbl)
            n54 = local read "Z_axis"() -> (w134:dbl)
            n55 = event shown="[23] \"Galvo Stop\": Value Change" {
              selector: _ -> [_ _ _ _ _ _ _ _ _ _ _ _ _ _ _ _ _ _ _ _ _ _ _ _]
              dyn-events: _ -> [_ _ _ _ _ _ _ _ _ _ _ _ _ _ _ _ _ _ _ _ _ _ _ _]
              timeout: 0 -> [_ _ _ _ _ _ _ _ _ _ _ _ _ _ _ _ _ _ _ _ _ _ _ _]
              tunnel: [States."CMOS live" States."CMOS live" States."CMOS live" States."CMOS live" States."CMOS live" States."CMOS live" States."CMOS live" States."CMOS live" States."CMOS live" States."CMOS live" States."CMOS live" States."CMOS live" States."CMOS live" States."CMOS live" States."Shut down" States."CMOS live" States."CMOS live" States."CMOS live" States."CMOS live" States."CMOS live" States."CMOS live" States."CMOS live" States."CMOS live" States."CMOS live"] -> w154
              tunnel: w153 -> [w194 w291 w333 w602 w625 w650 w673 w698 w722 w742 w743 w765 w779 w787 w819 w866 w936 w958 w969 w980 w991 w1002 w1004 w1211]
              tunnel: [w193 w291 w332 w602 w625 w650 w673 w698 w722 w742 w743 w759 w779 w787 w819 w838 w937 w958 w969 w980 w991 w1002 w1035 w1211] -> w152
              tunnel: w148 -> [w192 _ w331 _ _ _ _ _ _ _ w752 _ _ _ _ w863 _ _ _ _ _ _ w1006 _]
              tunnel: w150 -> [w191 _ _ _ _ _ _ _ _ _ _ _ _ _ _ _ _ _ _ _ _ _ _ _]
              tunnel: w149 -> [w190 _ w330 _ _ _ _ _ _ _ w745 _ _ _ _ w862 _ _ _ _ _ _ w1007 _]
              tunnel: [w188 w290 w342 w601 w624 w649 w672 w697 w721 w741 w756 w775 w781 w789 w818 w868 w940 w957 w968 w979 w990 w1001 w1065 w1217] -> w147
              tunnel: w146 -> [w188 w290 w342 w601 w624 w649 w672 w697 w721 w741 w756 w775 _ w789 w818 w868 w940 w957 w968 w979 w990 w1001 w1065 w1217]
              tunnel: [w189 w289 w328 w600 w623 w648 w671 w696 w720 w740 w755 w774 w780 w792 w817 w861 w935 w946 w967 w978 w989 w1000 w1064 w1216] -> w145
              tunnel: w144 -> [w189 w289 w328 w600 w623 w648 w671 w696 w720 w740 w755 w774 w780 _ w817 w861 w935 w946 w967 w978 w989 w1000 w1064 w1216]
              tunnel: w143 -> [_ _ _ _ _ _ _ _ _ _ _ _ _ w791 _ _ _ _ _ _ _ _ _ _]
              tunnel: w142 -> [_ _ _ _ _ _ _ _ _ _ _ _ _ _ _ w837 _ _ _ _ _ _ _ _]
              tunnel: w142 -> [w185 w285 w334 w597 w619 w642 w666 w689 w714 w733 _ _ _ _ _ w859 w924 _ _ _ _ _ _ _]
              tunnel: [w187 w288 w341 w599 w622 w647 w670 w695 w719 w739 w754 w760 w778 w786 w816 w822 w939 w956 w966 w977 w988 w999 w1034 w1213] -> w140
              tunnel: w141 -> [w187 w288 w341 w599 w622 w647 w670 w695 w719 w739 w754 w767 w778 w786 w816 w822 w939 w956 w966 w977 w988 w999 w1066 w1213]
              tunnel: [w161 w287 w339 w598 w621 w646 w669 w694 w718 w738 w753 w773 w777 w785 w815 w821 w901 w944 w963 w972 w984 w995 w1008 w1215] -> w139
              tunnel: w138 -> [w161 w287 w339 w598 w621 w646 w669 w694 w718 w738 w753 w773 w777 w785 w815 w821 w901 _ w962 w973 w985 w996 w1008 w1215]
              tunnel: w137 -> [_ _ _ w589 w614 w637 w662 _ _ _ _ _ _ _ _ _ _ _ _ _ _ _ _ _]
              tunnel: w136 -> [_ _ _ w592 w617 _ _ _ _ _ _ _ _ _ _ _ _ _ _ _ _ _ _ _]
              tunnel: w135 -> [_ _ _ _ _ w639 w664 _ _ _ _ _ _ _ _ _ _ _ _ _ _ _ _ _]
              tunnel: w134 -> [_ _ _ _ _ _ _ w686 w710 _ _ _ _ _ _ _ _ _ _ _ _ _ _ _]
              tunnel: w133 -> [_ _ _ _ _ _ _ w690 w713 _ _ _ _ _ _ _ _ _ _ _ _ _ _ _]
              event Timeout {
                w172 = 2
                # "By default when clicking the RUN button, the camera will automatically stream images in secquence. After changing any of the instrument parameters, the VI will jump back to \"CMOS live\" state and into the \"Timeout\" event."
                n56 = event-data() -> ()  [unwired: 1 in, 3 out]
                n57 = Unbundle(w185) -> ("Device Z"=w175:refnum<k24>, "Device X"=w174:refnum<k24>, "Device Y"=w173:refnum<k24>)
                n58 = Unbundle By Name(w161) -> ("Laser X"=w169:dbl, "Laser Y"=w168:dbl)
                n59 = Unbundle By Name("Box") -> ("Width"=w163:dbl, "Height"=w162:dbl)
                n60 = Quotient & Remainder(x=w191, y=10) -> (x-y*floor(x/y)=w197:i32)  [unwired: 1 out]
                n61 = invoke class="KCubeDCServo" method="GetPositionCounter"(reference=w175) -> ("GetPositionCounter"=w184:i32)  [unwired: 2 in, 2 out]
                n62 = invoke class="KCubeDCServo" method="GetPositionCounter"(reference=w174) -> ("GetPositionCounter"=w183:i32)  [unwired: 2 in, 2 out]
                n63 = invoke class="KCubeDCServo" method="GetPositionCounter"(reference=w173) -> ("GetPositionCounter"=w182:i32)  [unwired: 2 in, 2 out]
                n64 = Quotient & Remainder(x=w191, y=5) -> (x-y*floor(x/y)=w200:i32)  [unwired: 1 out]
                n65 = Equal To 0?(x=w197) -> (x = 0?=w195:bool)
                n66 = Equal To 0?(x=w200) -> (x = 0?=w199:bool)
                n67 = Divide(x=w163, y=w172) -> (x/y=w167:dbl)
                n68 = Subtract(x=w169, y=w167) -> (x-y=w165:dbl)
                n69 = Divide(x=w162, y=w172) -> (x/y=w166:dbl)
                n70 = Subtract(x=w168, y=w166) -> (x-y=w164:dbl)
                n71 = Add(x=w166, y=w168) -> (x+y=w170:dbl)
                n72 = Add(x=w169, y=w167) -> (x+y=w171:dbl)
                n73 = Divide(x=w184, y=34304) -> (x/y=→"Z_axis":dbl)
                n74 = Divide(x=w183, y=34304) -> (x/y=→"X_axis":dbl)
                n75 = Divide(x=w182, y=34304) -> (x/y=→"Y_axis":dbl)
                n76 = flat-sequence {
                  tunnel: w192 -> [w252]
                  tunnel: w194 -> [w251]
                  tunnel: [w250] -> w193
                  tunnel: [w249] -> w156
                  tunnel: w190 -> [w271]
                  tunnel: w189 -> [w263]
                  tunnel: w161 -> [w259]
                  tunnel: w158 -> [w258]
                  tunnel: [w257] -> w157
                  tunnel: w156 -> [w253]
                  frame #0 {
                    n77 = call "GetActImgMem.vi"("error in"=w251, "Camera Handle In"=w252) -> ("error out"=w250:errorcluster, "Image Memory Out"=w249:u8[])  [unwired: 6 in, 2 out]
                  }
                  frame #1 {
                    # "Display Image"
                    n78 = Unbundle(w271) -> ("Height"=w270:i32, "Width"=w269:i32)
                    n79 = Reshape Array(w253, w270, w269) -> (w268:u8[][])
                    n80 = call <vilib>:"Flatten Pixmap.vi"("colors"=u32[] [0, 65793, 131586, 197379, 263172, 328965, 394758, 460551, 526344, 592137, 657930, 723723, 789516, 855309, 921102, 986895, 1052688, 1118481, 1184274, 1250067, 1315860, 1381653, 1447446, 1513239, 1579032, 1644825, 1710618, 1776411, 1842204, 1907997, 1973790, 2039583, 2105376, 2171169, 2236962, 2302755, 2368548, 2434341, 2500134, 2565927, 2631720, 2697513, 2763306, 2829099, 2894892, 2960685, 3026478, 3092271, 3158064, 3223857, 3289650, 3355443, 3421236, 3487029, 3552822, 3618615, 3684408, 3750201, 3815994, 3881787, 3947580, 4013373, 4079166, 4144959, 4210752, 4276545, 4342338, 4408131, 4473924, 4539717, 4605510, 4671303, 4737096, 4802889, 4868682, 4934475, 5000268, 5066061, 5131854, 5197647, 5263440, 5329233, 5395026, 5460819, 5526612, 5592405, 5658198, 5723991, 5789784, 5855577, 5921370, 5987163, 6052956, 6118749, 6184542, 6250335, 6316128, 6381921, 6447714, 6513507, 6579300, 6645093, 6710886, 6776679, 6842472, 6908265, 6974058, 7039851, 7105644, 7171437, 7237230, 7303023, 7368816, 7434609, 7500402, 7566195, 7631988, 7697781, 7763574, 7829367, 7895160, 7960953, 8026746, 8092539, 8158332, 8224125, 8289918, 8355711, 8421504, 8487297, 8553090, 8618883, 8684676, 8750469, 8816262, 8882055, 8947848, 9013641, 9079434, 9145227, 9211020, 9276813, 9342606, 9408399, 9474192, 9539985, 9605778, 9671571, 9737364, 9803157, 9868950, 9934743, 10000536, 10066329, 10132122, 10197915, 10263708, 10329501, 10395294, 10461087, 10526880, 10592673, 10658466, 10724259, 10790052, 10855845, 10921638, 10987431, 11053224, 11119017, 11184810, 11250603, 11316396, 11382189, 11447982, 11513775, 11579568, 11645361, 11711154, 11776947, 11842740, 11908533, 11974326, 12040119, 12105912, 12171705, 12237498, 12303291, 12369084, 12434877, 12500670, 12566463, 12632256, 12698049, 12763842, 12829635, 12895428, 12961221, 13027014, 13092807, 13158600, 13224393, 13290186, 13355979, 13421772, 13487565, 13553358, 13619151, 13684944, 13750737, 13816530, 13882323, 13948116, 14013909, 14079702, 14145495, 14211288, 14277081, 14342874, 14408667, 14474460, 14540253, 14606046, 14671839, 14737632, 14803425, 14869218, 14935011, 15000804, 15066597, 15132390, 15198183, 15263976, 15329769, 15395562, 15461355, 15527148, 15592941, 15658734, 15724527, 15790320, 15856113, 15921906, 15987699, 16053492, 16119285, 16185078, 16250871, 16316664, 16382457, 16448250, 16514043, 16579836, 16645629, 16711422, 0] ("output array 2"), "8-bit pixmap"=w268) -> ("image data"=w267:T33)  [unwired: 9 in]
                    n81 = call <vilib>:"Draw Flattened Pixmap.vi"("image data"=w267) -> ("new picture"=w264:picture)  [unwired: 8 in]
                    n82 = call <vilib>:"Draw Rectangle.vi"("picture"=w264, "rect"=w263, "color(black)"=u32 16318226) -> ("new picture"=w262:picture)  [unwired: 6 in]
                    n83 = local read "Boolean"() -> (w260:bool)
                    n84 = case shown="True" w260 {
                      tunnel: w262 -> [w272 w275]
                      tunnel: [w272 w278] -> w261
                      tunnel: w259 -> [_ w277]
                      tunnel: w258 -> [_ w276]
                      frame False {
                      }
                      frame True {
                        n85 = call <vilib>:"Draw Rectangle.vi"("picture"=w275, "rect"=w276, "color(black)"=u32 6618880) -> ("new picture"=w274:picture)  [unwired: 6 in]
                        n86 = To Word Integer(number=w277) -> (16bit integer=w279:cluster{"Laser X":i16, "Laser Y":i16})
                        n87 = call <vilib>:"Draw Point.vi"("picture"=w274, "point(x,y)"=w279, "color(black)"=u32 16711680, "pen"=T27 {"Width"=5, "Style"=enum."Solid"}) -> ("new picture"=w278:picture)  [unwired: 5 in]
                      }
                    }
                    "Live video" <- w261
                    n88 = local read "Frame rate"() -> (w254:dbl)
                    n89 = Reciprocal(x=w254) -> (1/x=w256:dbl)
                    n90 = Multiply(x=w256, y=1000) -> (x*y=w257:dbl)
                  }
                }
                n91 = Bundle By Name(cluster=T21 {"left"=0, "top"=0, "right"=0, "bottom"=0} ("rect"), "left"=w165, "top"=w164, "right"=w171, "bottom"=w170) -> (w158:T21)
                n92 = case shown="True" w199 {
                  tunnel: w192 -> [_ w235]
                  frame False {
                  }
                  frame True {
                    # "Set Slider Range"
                    n93 = call "GetFramesPerSecond.vi"("Camera Handle In"=w235) -> ("FPS"=→"FPS":dbl)  [unwired: 8 in, 2 out]
                    n94 = call "GetExposureRange.vi"("Camera Handle In"=w235) -> ("max"=w245:dbl, "min"=w246:dbl, "intervall"=w244:dbl)  [unwired: 6 in, 2 out]
                    n95 = Bundle("min"=w246, "max"=w245, "intervall"=w244) -> (w247:cluster{"min":dbl, "max":dbl, "intervall":dbl})  [unwired: 1 in]
                    n96 = property on="Exposure time (ms)" class="Schieberegler (strikt)"("Scale.Minimum"=w246, "Scale.Maximum"=w245, "Scale.Increment"=w244) -> ()  [unwired: 2 in, 2 out]
                    n97 = property on="Exposure time (ms)" class="Schieberegler (strikt)"("Data Range"=w247) -> ()  [unwired: 2 in, 2 out]
                    n98 = call "GetFrameTimeRange.vi"("Camera Handle In"=w235) -> ("max"=w241:dbl, "min"=w240:dbl, "interval"=w237:dbl)  [unwired: 6 in, 2 out]
                    n99 = Reciprocal(x=w241) -> (1/x=w239:dbl)
                    n100 = Reciprocal(x=w240) -> (1/x=w238:dbl)
                    n101 = property on="Frame rate" class="Schieberegler (strikt)"("Minimum"=w239, "Maximum"=w238, "Increment"=w237) -> ()  [unwired: 2 in, 2 out]
                    n102 = property on="Frame rate" class="Schieberegler (strikt)"("Scale.Minimum"=w239, "Scale.Maximum"=w238, "Scale.Increment"=w237) -> ()  [unwired: 2 in, 2 out]
                    n103 = call "GetPixelClockRange.vi"("Camera Handle In"=w235) -> ("Max"=w243:i32, "Min"=w242:i32)  [unwired: 7 in, 2 out]
                    n104 = property on="Pixel clock" class="Schieberegler (strikt)"("Scale.Minimum"=w242, "Scale.Maximum"=w243) -> ()  [unwired: 2 in, 2 out]
                    n105 = property on="Pixel clock" class="Schieberegler (strikt)"("Minimum"=w242, "Maximum"=w243) -> ()  [unwired: 2 in, 2 out]
                    n106 = call "SetAOI.vi"("Camera Handle In"=w235, "Mode"=32771) -> ("Width Out"=→"Width":i32, "Height Out"=→"Height":i32)  [unwired: 8 in, 4 out]
                  }
                }
                n107 = case shown="True" w195 {
                  tunnel: w192 -> [_ w204]
                  frame False {
                  }
                  frame True {
                    # "Set Exposure time, Pixelclock\nand Framerate"
                    n108 = call "ThorSetExposureTime.vi"("Mode"=u16 32900, "Exposure Time"="Exposure time (ms)", "Camera Handle In"=w204) -> ()  [unwired: 6 in, 3 out]
                    n109 = call "SetFrameRate.vi"("FPS"="Frame rate", "Camera Handle In"=w204) -> ()  [unwired: 7 in, 3 out]
                    n110 = call "SetPixelClock.vi"("Mode"=32770, "Pixel Clock"="Pixel clock", "Camera Handle In"=w204) -> ()  [unwired: 6 in, 3 out]
                    n111 = call "SetAutoParameter.vi"("enable"="Autogain", "Param"=34816, "Camera Handle In"=w204) -> ("Camera Handle Out"=w212:u32)  [unwired: 6 in, 2 out]
                    n112 = case shown="True" "Edge Filter Enable / Disable" {
                      tunnel: w204 -> [w214 w217]
                      frame False {
                        n113 = call "SetEdgeEnhancement.vi"("Mode"=0, "Camera Handle In"=w214) -> ()  [unwired: 8 in, 2 out]
                      }
                      frame True {
                        n114 = call "SetEdgeEnhancement.vi"("Mode"="Edge Filter", "Camera Handle In"=w217) -> ()  [unwired: 8 in, 2 out]
                      }
                    }
                    n115 = case shown="False" "Autogain" {
                      tunnel: w212 -> [w228 w231]
                      frame False {
                        # "Set Master Gain"
                        n116 = call "SetHardwareGain.vi"("Master Gain"="Master Gain", "Camera Handle In"=w228) -> ()  [unwired: 7 in, 3 out]
                      }
                      frame True {
                        w230 = 32768 items=["IS_GET_MASTER_GAIN"=32768]
                        # "On active AutoGain\nset Master Gain Slider Value"
                        n117 = call "SetHardwareGain.vi"("Mode"=w230, "Camera Handle In"=w231) -> ("Value"=w232:i32)  [unwired: 7 in, 2 out]
                        n118 = property on="Master Gain" class="Slide (strict)"("Value"=w232) -> ()  [unwired: 2 in, 2 out]
                      }
                    }
                    n119 = case shown="False" "Hotpixel correction 2" {
                      tunnel: w204 -> [w225 w227]
                      frame False {
                        n120 = call "SetHotPixelCorrection.vi"("Mode"=0, "Camera Handle In"=w225) -> ()  [unwired: 7 in, 3 out]
                      }
                      frame True {
                        n121 = call "SetHotPixelCorrection.vi"("Mode"=2, "Camera Handle In"=w227) -> ()  [unwired: 7 in, 3 out]
                      }
                    }
                    n122 = case shown="True" "Blacklevel compensation" {
                      tunnel: w204 -> [w220 w223]
                      tunnel: "Blacklevel Offset" -> [w218 w221]
                      frame False {
                        n123 = call "SetBlCompensation.vi"("Mode"=0, "offset"=w218, "Camera Handle In"=w220) -> ()  [unwired: 6 in, 3 out]
                      }
                      frame True {
                        n124 = call "SetBlCompensation.vi"("Mode"=1, "offset"=w221, "Camera Handle In"=w223) -> ()  [unwired: 6 in, 3 out]
                      }
                    }
                  }
                }
                n125 = Wait Until Next ms Multiple(millisecond multiple=w157) -> ()  [unwired: 1 out]
              }
              event "Reset": Value Change {
                n126 = event-data() -> ()  [unwired: 1 in, 6 out]
                n127 = Unbundle(w285) -> ("Device Z"=w284:refnum<k24>, "Device X"=w283:refnum<k24>, "Device Y"=w282:refnum<k24>)
                n128 = stacked-sequence {
                  tunnel: w284 -> [w295 _ _ _ _ w317 w322 w325 _]
                  tunnel: w282 -> [_ _ w301 _ w313 _ _ w324 _]
                  tunnel: w283 -> [_ w297 _ w308 _ _ _ w323 _]
                  frame #0 {
                    # "Move Z to maxinum"
                    n129 = invoke class="KCubeDCServo" method="MoveTo"(reference=w295, "position"=12.0, "waitTimeout"=0) -> ()  [unwired: 2 in, 5 out]
                    n130 = Wait (ms)(milliseconds to wait=u32 10000) -> ()  [unwired: 1 out]
                  }
                  frame #1 {
                    # "Make X home"
                    n131 = invoke class="KCubeDCServo" method="Home"(reference=w297, "waitTimeout"=0) -> (reference out=w296:refnum<k24>)  [unwired: 2 in, 3 out]
                    n132 = invoke class="KCubeDCServo" method="ClearDeviceExceptions"(reference=w296) -> ()  [unwired: 2 in, 3 out]
                    n133 = Wait (ms)(milliseconds to wait=u32 30000) -> ()  [unwired: 1 out]
                  }
                  frame #2 {
                    # "Make Y home"
                    n134 = invoke class="KCubeDCServo" method="Home"(reference=w301, "waitTimeout"=0) -> (reference out=w300:refnum<k24>)  [unwired: 2 in, 3 out]
                    n135 = invoke class="KCubeDCServo" method="ClearDeviceExceptions"(reference=w300) -> ()  [unwired: 2 in, 3 out]
                    n136 = Wait (ms)(milliseconds to wait=u32 30000) -> ()  [unwired: 1 out]
                  }
                  frame #3 {
                    # "Move X to center"
                    n137 = invoke class="KCubeDCServo" method="MoveTo"(reference=w308, "position"=7.0, "waitTimeout"=0) -> (reference out=w304:refnum<k24>)  [unwired: 2 in, 4 out]
                    n138 = invoke class="KCubeDCServo" method="ClearDeviceExceptions"(reference=w304) -> ()  [unwired: 2 in, 3 out]
                    n139 = Wait (ms)(milliseconds to wait=u32 5000) -> ()  [unwired: 1 out]
                  }
                  frame #4 {
                    # "Move Y to center"
                    n140 = invoke class="KCubeDCServo" method="MoveTo"(reference=w313, "position"=7.0, "waitTimeout"=0) -> (reference out=w309:refnum<k24>)  [unwired: 2 in, 4 out]
                    n141 = invoke class="KCubeDCServo" method="ClearDeviceExceptions"(reference=w309) -> ()  [unwired: 2 in, 3 out]
                    n142 = Wait (ms)(milliseconds to wait=u32 5000) -> ()  [unwired: 1 out]
                  }
                  frame #5 {
                    # "Z: home"
                    n143 = invoke class="KCubeDCServo" method="Home"(reference=w317, "waitTimeout"=0) -> (reference out=w314:refnum<k24>)  [unwired: 2 in, 3 out]
                    n144 = invoke class="KCubeDCServo" method="ClearDeviceExceptions"(reference=w314) -> ()  [unwired: 2 in, 3 out]
                    n145 = Wait (ms)(milliseconds to wait=u32 40000) -> ()  [unwired: 1 out]
                  }
                  frame #6 {
                    # "Move satge along Z about 0.5mm"
                    n146 = invoke class="KCubeDCServo" method="MoveTo"(reference=w322, "position"=4.5, "waitTimeout"=0) -> (reference out=w318:refnum<k24>)  [unwired: 2 in, 4 out]
                    n147 = Wait (ms)(milliseconds to wait=u32 5000) -> ()  [unwired: 1 out]
                    n148 = invoke class="KCubeDCServo" method="ClearDeviceExceptions"(reference=w318) -> ()  [unwired: 2 in, 3 out]
                  }
                  frame #7 {
                    n149 = invoke class="KCubeDCServo" method="ClearDeviceExceptions"(reference=w323) -> ()  [unwired: 2 in, 3 out]
                    n150 = invoke class="KCubeDCServo" method="ClearDeviceExceptions"(reference=w324) -> ()  [unwired: 2 in, 3 out]
                    n151 = invoke class="KCubeDCServo" method="ClearDeviceExceptions"(reference=w325) -> ()  [unwired: 2 in, 3 out]
                  }
                  frame #8 {
                    n152 = call "Display Message to User"("Enable"=TRUE, "Message"="Reset has been completed!!") -> ()  [unwired: 8 in, 2 out]
                  }
                }
              }
              event "Scan": Value Change {
                n153 = event-data() -> ()  [unwired: 1 in, 6 out]
                n154 = Unbundle By Name(w328) -> ("left"=w338:i16, "top"=w336:i16, "right"=w337:i16, "bottom"=w335:i16)
                n155 = stacked-sequence {
                  tunnel: w339 -> [_ w375 _ _]
                  tunnel: w338 -> [_ w357 w408 _]
                  tunnel: w337 -> [_ _ w409 _]
                  tunnel: w336 -> [_ w356 w401 _]
                  tunnel: w335 -> [_ _ w402 _]
                  tunnel: w334 -> [_ w360 w400 _]
                  tunnel: w333 -> [_ w359 _ _]
                  tunnel: [_ w358 _ _] -> w332
                  tunnel: w331 -> [w343 _ w399 _]
                  tunnel: w330 -> [w344 _ w398 _]
                  tunnel: "Save Path" -> [w346 _ w397 _]
                  frame #0 {
                    n156 = Unbundle(w344) -> ("Height"=w349:i32, "Width"=w348:i32)
                    n157 = Build Path(base path=w346, name or relative path="Crop_Area.png") -> (appended path=w350:path)
                    n158 = call "GetActImgMem.vi"("Camera Handle In"=w343) -> ("Image Memory Out"=w353:u8[])  [unwired: 7 in, 3 out]
                    n159 = Reshape Array(w353, w349, w348) -> (w354:u8[][])
                    n160 = call <vilib>:"Flatten Pixmap.vi"("colors"=u32[] [0, 65793, 131586, 197379, 263172, 328965, 394758, 460551, 526344, 592137, 657930, 723723, 789516, 855309, 921102, 986895, 1052688, 1118481, 1184274, 1250067, 1315860, 1381653, 1447446, 1513239, 1579032, 1644825, 1710618, 1776411, 1842204, 1907997, 1973790, 2039583, 2105376, 2171169, 2236962, 2302755, 2368548, 2434341, 2500134, 2565927, 2631720, 2697513, 2763306, 2829099, 2894892, 2960685, 3026478, 3092271, 3158064, 3223857, 3289650, 3355443, 3421236, 3487029, 3552822, 3618615, 3684408, 3750201, 3815994, 3881787, 3947580, 4013373, 4079166, 4144959, 4210752, 4276545, 4342338, 4408131, 4473924, 4539717, 4605510, 4671303, 4737096, 4802889, 4868682, 4934475, 5000268, 5066061, 5131854, 5197647, 5263440, 5329233, 5395026, 5460819, 5526612, 5592405, 5658198, 5723991, 5789784, 5855577, 5921370, 5987163, 6052956, 6118749, 6184542, 6250335, 6316128, 6381921, 6447714, 6513507, 6579300, 6645093, 6710886, 6776679, 6842472, 6908265, 6974058, 7039851, 7105644, 7171437, 7237230, 7303023, 7368816, 7434609, 7500402, 7566195, 7631988, 7697781, 7763574, 7829367, 7895160, 7960953, 8026746, 8092539, 8158332, 8224125, 8289918, 8355711, 8421504, 8487297, 8553090, 8618883, 8684676, 8750469, 8816262, 8882055, 8947848, 9013641, 9079434, 9145227, 9211020, 9276813, 9342606, 9408399, 9474192, 9539985, 9605778, 9671571, 9737364, 9803157, 9868950, 9934743, 10000536, 10066329, 10132122, 10197915, 10263708, 10329501, 10395294, 10461087, 10526880, 10592673, 10658466, 10724259, 10790052, 10855845, 10921638, 10987431, 11053224, 11119017, 11184810, 11250603, 11316396, 11382189, 11447982, 11513775, 11579568, 11645361, 11711154, 11776947, 11842740, 11908533, 11974326, 12040119, 12105912, 12171705, 12237498, 12303291, 12369084, 12434877, 12500670, 12566463, 12632256, 12698049, 12763842, 12829635, 12895428, 12961221, 13027014, 13092807, 13158600, 13224393, 13290186, 13355979, 13421772, 13487565, 13553358, 13619151, 13684944, 13750737, 13816530, 13882323, 13948116, 14013909, 14079702, 14145495, 14211288, 14277081, 14342874, 14408667, 14474460, 14540253, 14606046, 14671839, 14737632, 14803425, 14869218, 14935011, 15000804, 15066597, 15132390, 15198183, 15263976, 15329769, 15395562, 15461355, 15527148, 15592941, 15658734, 15724527, 15790320, 15856113, 15921906, 15987699, 16053492, 16119285, 16185078, 16250871, 16316664, 16382457, 16448250, 16514043, 16579836, 16645629, 16711422, 0] ("output array 2"), "8-bit pixmap"=w354) -> ("image data"=w351:T33)  [unwired: 9 in]
                    n161 = Wait (ms)(milliseconds to wait=u32 300) -> ()  [unwired: 1 out]
                    n162 = call <vilib>:"Write PNG File.vi"("image data"=w351, "path to PNG file"=w350) -> ()  [unwired: 8 in, 2 out]
                  }
                  frame #1 {
                    n163 = Unbundle By Name(w375) -> ("Laser X"=w367:dbl, "Laser Y"=w366:dbl)
                    n164 = Subtract(x=w367, y=w357) -> (x-y=w365:dbl)
                    n165 = Subtract(x=w366, y=w356) -> (x-y=w363:dbl)
                    n166 = Divide(x=0.0877, y=1000.0) -> (x/y=w364:dbl)
                    n167 = Multiply(x=w364, y=w365) -> (x*y=w362:dbl)
                    n168 = Multiply(x=w364, y=w363) -> (x*y=w361:dbl)
                    n169 = call "StageReadPos.vi"("error in (no error)"=w359, "Stage Select"=StageSelect."X axis", "Device In"=w360) -> ("error out"=w374:errorcluster, "CurrentPosition"=w372:dbl)  [unwired: 7 in]
                    n170 = call "StageReadPos.vi"("error in (no error)"=w359, "Stage Select"=StageSelect."Y axis", "Device In"=w360) -> ("error out"=w370:errorcluster, "CurrentPosition"=w369:dbl)  [unwired: 7 in]
                    n171 = stacked-sequence {
                      tunnel: w374 -> [w394 _]
                      tunnel: w372 -> [w392 _]
                      tunnel: [w390 _] -> w368
                      tunnel: w362 -> [w389 _]
                      tunnel: w360 -> [w388 _]
                      frame #0 {
                        n172 = Add(x=w389, y=w392) -> (x+y=w391:dbl)
                        n173 = call "StageToPos.vi"("error in (no error)"=w394, "Move to pos"=w391, "Stage Select"=StageSelect."X axis", "Device In"=w388) -> ("error out"=w390:errorcluster)  [unwired: 7 in]
                      }
                      frame #1 {
                        n174 = Wait (ms)(milliseconds to wait=u32 400) -> ()  [unwired: 1 out]
                      }
                    }
                    n175 = stacked-sequence {
                      tunnel: w370 -> [w385 _]
                      tunnel: w369 -> [w384 _]
                      tunnel: w368 -> [w382 _]
                      tunnel: w361 -> [w380 _]
                      tunnel: w360 -> [w379 _]
                      tunnel: [w378 _] -> w358
                      frame #0 {
                        n176 = Add(x=w380, y=w384) -> (x+y=w383:dbl)
                        n177 = call "StageToPos.vi"("error in (no error)"=w385, "Move to pos"=w383, "Stage Select"=StageSelect."Y axis", "Device In"=w379) -> ("error out"=w381:errorcluster)  [unwired: 7 in]
                        n178 = Merge Errors(w382, w381) -> (w378:errorcluster)
                      }
                      frame #1 {
                        n179 = Wait (ms)(milliseconds to wait=u32 400) -> ()  [unwired: 1 out]
                      }
                    }
                    n180 = Wait (ms)(milliseconds to wait=u32 100) -> ()  [unwired: 1 out]
                  }
                  frame #2 {
                    n181 = Subtract(x=w402, y=w401) -> (x-y=w404:i16)
                    n182 = Subtract(x=w409, y=w408) -> (x-y=w407:i16)
                    n183 = Divide(x=w404, y=i16 50) -> (x/y=w396:dbl)
                    n184 = Divide(x=w407, y=i16 50) -> (x/y=w405:dbl)
                    n185 = for {
                      N: w396 -> [w416]
                      tunnel: w405 -> [w410]
                      tunnel: w400 -> [w420]
                      tunnel: w399 -> [w419]
                      tunnel: w398 -> [w418]
                      tunnel: w397 -> [w417]
                      i -> [w413]
                      n186 = Round Toward -Infinity(1:w410) -> (0:→"Total_Frame_X":dbl)
                      n187 = Increment(x=w413) -> (x+1=→"Frame_Y":i32)
                      n188 = Divide(x=w413, y=2) -> (x/y=w425:dbl)
                      n189 = Round Toward -Infinity(1:w425) -> (0:w422:dbl)
                      n190 = Round Toward +Infinity(x=w425) -> (ceil(x): smallest int >= x=w423:dbl)
                      n191 = Equal?(x=w423, y=w422) -> (x = y?=w421:bool)
                      n192 = stacked-sequence {
                        tunnel: w421 -> [_ w438 w490]
                        tunnel: w410 -> [_ _ w489]
                        tunnel: w420 -> [w435 _ w488]
                        tunnel: w419 -> [_ w439 w487]
                        tunnel: w418 -> [_ w440 w486]
                        tunnel: w417 -> [_ w441 w485]
                        tunnel: w413 -> [_ w437 w484]
                        tunnel: w410 -> [_ w436 w483]
                        tunnel: [_ _ w482] -> w415
                        frame #0 {
                          w433 = 1 items=["Forward"=1, "Backward"=2] ("direction")
                          n193 = Unbundle By Name(w435) -> ("Device Y"=w434:refnum<k24>)  [unwired: 2 out]
                          n194 = Divide(x=0.0877 ("y"), y=1000.0) -> (x/y=w426:dbl)
                          n195 = Multiply(x=50.0, y=w426) -> (x*y=w429:dbl)
                          n196 = invoke class="KCubeDCServo" method="MoveRelative"(reference=w434, "direction"=w433, "stepSize"=w429, "waitTimeout"=0) -> ()  [unwired: 2 in, 6 out]
                          n197 = Wait (ms)(milliseconds to wait=u32 300) -> ()  [unwired: 1 out]
                        }
                        frame #1 {
                          n198 = case shown="False" w438 {
                            tunnel: w441 -> [w448 w467]
                            tunnel: w440 -> [w446 w466]
                            tunnel: w439 -> [w447 w465]
                            tunnel: w437 -> [w444 w463]
                            tunnel: w436 -> [w443 _]
                            frame False {
                              n199 = Round Toward -Infinity(1:w443) -> (0:w442:dbl)
                              n200 = Increment(x=w444) -> (x+1=w449:i32)
                              n201 = Number To Decimal String(number=w442) -> (decimal integer string=w445:string)  [unwired: 1 in]
                              n202 = Number To Decimal String(number=w449) -> (decimal integer string=w454:string)  [unwired: 1 in]
                              n203 = Concatenate Strings("x" ("string"), w445, "_y" ("string"), w454, ".png" ("string")) -> (w458:string)
                              n204 = Unbundle(w446) -> ("Height"=w452:i32, "Width"=w451:i32)
                              n205 = Build Path(base path=w448, name or relative path=w458) -> (appended path=w453:path)
                              n206 = call "GetActImgMem.vi"("Camera Handle In"=w447) -> ("Image Memory Out"=w461:u8[])  [unwired: 7 in, 3 out]
                              n207 = Reshape Array(w461, w452, w451) -> (w462:u8[][])
                              n208 = call <vilib>:"Flatten Pixmap.vi"("colors"=u32[] [0, 65793, 131586, 197379, 263172, 328965, 394758, 460551, 526344, 592137, 657930, 723723, 789516, 855309, 921102, 986895, 1052688, 1118481, 1184274, 1250067, 1315860, 1381653, 1447446, 1513239, 1579032, 1644825, 1710618, 1776411, 1842204, 1907997, 1973790, 2039583, 2105376, 2171169, 2236962, 2302755, 2368548, 2434341, 2500134, 2565927, 2631720, 2697513, 2763306, 2829099, 2894892, 2960685, 3026478, 3092271, 3158064, 3223857, 3289650, 3355443, 3421236, 3487029, 3552822, 3618615, 3684408, 3750201, 3815994, 3881787, 3947580, 4013373, 4079166, 4144959, 4210752, 4276545, 4342338, 4408131, 4473924, 4539717, 4605510, 4671303, 4737096, 4802889, 4868682, 4934475, 5000268, 5066061, 5131854, 5197647, 5263440, 5329233, 5395026, 5460819, 5526612, 5592405, 5658198, 5723991, 5789784, 5855577, 5921370, 5987163, 6052956, 6118749, 6184542, 6250335, 6316128, 6381921, 6447714, 6513507, 6579300, 6645093, 6710886, 6776679, 6842472, 6908265, 6974058, 7039851, 7105644, 7171437, 7237230, 7303023, 7368816, 7434609, 7500402, 7566195, 7631988, 7697781, 7763574, 7829367, 7895160, 7960953, 8026746, 8092539, 8158332, 8224125, 8289918, 8355711, 8421504, 8487297, 8553090, 8618883, 8684676, 8750469, 8816262, 8882055, 8947848, 9013641, 9079434, 9145227, 9211020, 9276813, 9342606, 9408399, 9474192, 9539985, 9605778, 9671571, 9737364, 9803157, 9868950, 9934743, 10000536, 10066329, 10132122, 10197915, 10263708, 10329501, 10395294, 10461087, 10526880, 10592673, 10658466, 10724259, 10790052, 10855845, 10921638, 10987431, 11053224, 11119017, 11184810, 11250603, 11316396, 11382189, 11447982, 11513775, 11579568, 11645361, 11711154, 11776947, 11842740, 11908533, 11974326, 12040119, 12105912, 12171705, 12237498, 12303291, 12369084, 12434877, 12500670, 12566463, 12632256, 12698049, 12763842, 12829635, 12895428, 12961221, 13027014, 13092807, 13158600, 13224393, 13290186, 13355979, 13421772, 13487565, 13553358, 13619151, 13684944, 13750737, 13816530, 13882323, 13948116, 14013909, 14079702, 14145495, 14211288, 14277081, 14342874, 14408667, 14474460, 14540253, 14606046, 14671839, 14737632, 14803425, 14869218, 14935011, 15000804, 15066597, 15132390, 15198183, 15263976, 15329769, 15395562, 15461355, 15527148, 15592941, 15658734, 15724527, 15790320, 15856113, 15921906, 15987699, 16053492, 16119285, 16185078, 16250871, 16316664, 16382457, 16448250, 16514043, 16579836, 16645629, 16711422, 0] ("output array 2"), "8-bit pixmap"=w462) -> ("image data"=w459:T33)  [unwired: 9 in]
                              n209 = Wait (ms)(milliseconds to wait=u32 300) -> ()  [unwired: 1 out]
                              n210 = call <vilib>:"Write PNG File.vi"("image data"=w459, "path to PNG file"=w453) -> ()  [unwired: 8 in, 2 out]
                            }
                            frame True {
                              n211 = Increment(x=w463) -> (x+1=w468:i32)
                              n212 = Number To Decimal String(number=w468) -> (decimal integer string=w473:string)  [unwired: 1 in]
                              n213 = Concatenate Strings("x" ("string"), "0" ("string"), "_y" ("string"), w473, ".png" ("string")) -> (w477:string)
                              n214 = Unbundle(w466) -> ("Height"=w471:i32, "Width"=w470:i32)
                              n215 = Build Path(base path=w467, name or relative path=w477) -> (appended path=w472:path)
                              n216 = call "GetActImgMem.vi"("Camera Handle In"=w465) -> ("Image Memory Out"=w480:u8[])  [unwired: 7 in, 3 out]
                              n217 = Reshape Array(w480, w471, w470) -> (w481:u8[][])
                              n218 = call <vilib>:"Flatten Pixmap.vi"("colors"=u32[] [0, 65793, 131586, 197379, 263172, 328965, 394758, 460551, 526344, 592137, 657930, 723723, 789516, 855309, 921102, 986895, 1052688, 1118481, 1184274, 1250067, 1315860, 1381653, 1447446, 1513239, 1579032, 1644825, 1710618, 1776411, 1842204, 1907997, 1973790, 2039583, 2105376, 2171169, 2236962, 2302755, 2368548, 2434341, 2500134, 2565927, 2631720, 2697513, 2763306, 2829099, 2894892, 2960685, 3026478, 3092271, 3158064, 3223857, 3289650, 3355443, 3421236, 3487029, 3552822, 3618615, 3684408, 3750201, 3815994, 3881787, 3947580, 4013373, 4079166, 4144959, 4210752, 4276545, 4342338, 4408131, 4473924, 4539717, 4605510, 4671303, 4737096, 4802889, 4868682, 4934475, 5000268, 5066061, 5131854, 5197647, 5263440, 5329233, 5395026, 5460819, 5526612, 5592405, 5658198, 5723991, 5789784, 5855577, 5921370, 5987163, 6052956, 6118749, 6184542, 6250335, 6316128, 6381921, 6447714, 6513507, 6579300, 6645093, 6710886, 6776679, 6842472, 6908265, 6974058, 7039851, 7105644, 7171437, 7237230, 7303023, 7368816, 7434609, 7500402, 7566195, 7631988, 7697781, 7763574, 7829367, 7895160, 7960953, 8026746, 8092539, 8158332, 8224125, 8289918, 8355711, 8421504, 8487297, 8553090, 8618883, 8684676, 8750469, 8816262, 8882055, 8947848, 9013641, 9079434, 9145227, 9211020, 9276813, 9342606, 9408399, 9474192, 9539985, 9605778, 9671571, 9737364, 9803157, 9868950, 9934743, 10000536, 10066329, 10132122, 10197915, 10263708, 10329501, 10395294, 10461087, 10526880, 10592673, 10658466, 10724259, 10790052, 10855845, 10921638, 10987431, 11053224, 11119017, 11184810, 11250603, 11316396, 11382189, 11447982, 11513775, 11579568, 11645361, 11711154, 11776947, 11842740, 11908533, 11974326, 12040119, 12105912, 12171705, 12237498, 12303291, 12369084, 12434877, 12500670, 12566463, 12632256, 12698049, 12763842, 12829635, 12895428, 12961221, 13027014, 13092807, 13158600, 13224393, 13290186, 13355979, 13421772, 13487565, 13553358, 13619151, 13684944, 13750737, 13816530, 13882323, 13948116, 14013909, 14079702, 14145495, 14211288, 14277081, 14342874, 14408667, 14474460, 14540253, 14606046, 14671839, 14737632, 14803425, 14869218, 14935011, 15000804, 15066597, 15132390, 15198183, 15263976, 15329769, 15395562, 15461355, 15527148, 15592941, 15658734, 15724527, 15790320, 15856113, 15921906, 15987699, 16053492, 16119285, 16185078, 16250871, 16316664, 16382457, 16448250, 16514043, 16579836, 16645629, 16711422, 0] ("output array 2"), "8-bit pixmap"=w481) -> ("image data"=w478:T33)  [unwired: 9 in]
                              n219 = Wait (ms)(milliseconds to wait=u32 300) -> ()  [unwired: 1 out]
                              n220 = call <vilib>:"Write PNG File.vi"("image data"=w478, "path to PNG file"=w472) -> ()  [unwired: 8 in, 2 out]
                            }
                          }
                        }
                        frame #2 {
                          n221 = case shown="False" w490 {
                            tunnel: w489 -> [w498 w547]
                            tunnel: w488 -> [w497 w546]
                            tunnel: w487 -> [w495 w545]
                            tunnel: w486 -> [w492 w544]
                            tunnel: w485 -> [w496 w543]
                            tunnel: w484 -> [w494 w542]
                            tunnel: w483 -> [w493 _]
                            tunnel: [w491 w541] -> w482
                            frame False {
                              n222 = for {
                                N: w498 -> [_]
                                tunnel: w497 -> [w505]
                                tunnel: w496 -> [w504]
                                tunnel: w495 -> [w503]
                                tunnel: w494 -> [w502]
                                tunnel: w493 -> [w501]
                                tunnel: w492 -> [w500]
                                tunnel: [w499] -> w491
                                i -> [w499]
                                n223 = stacked-sequence {
                                tunnel: w505 -> [_ w510 _]
                                tunnel: w504 -> [_ _ w529]
                                tunnel: w503 -> [_ _ w528]
                                tunnel: w502 -> [_ _ w523]
                                tunnel: w499 -> [_ _ w521]
                                tunnel: w501 -> [_ _ w520]
                                tunnel: w500 -> [_ _ w527]
                                frame #0 {
                                n224 = Wait (ms)(milliseconds to wait=u32 100) -> ()  [unwired: 1 out]
                                }
                                frame #1 {
                                w516 = 2 items=["Forward"=1, "Backward"=2] ("direction")
                                n225 = Unbundle By Name(w510) -> ("Device X"=w511:refnum<k24>)  [unwired: 2 out]
                                n226 = Divide(x=0.0877 ("y"), y=1000.0) -> (x/y=w508:dbl)
                                n227 = Multiply(x=50.0, y=w508) -> (x*y=w512:dbl)
                                n228 = invoke class="KCubeDCServo" method="MoveRelative"(reference=w511, "direction"=w516, "stepSize"=w512, "waitTimeout"=0) -> ()  [unwired: 2 in, 6 out]
                                n229 = Wait (ms)(milliseconds to wait=u32 450) -> ()  [unwired: 1 out]
                                }
                                frame #2 {
                                n230 = Round Toward -Infinity(1:w520) -> (0:w519:dbl)
                                n231 = Decrement(x=w519) -> (x-1=w518:dbl)
                                n232 = Subtract(x=w518, y=w521) -> (x-y=w517:dbl)
                                n233 = Increment(x=w523) -> (x+1=w522:i32)
                                n234 = Number To Decimal String(number=w517) -> (decimal integer string=w532:string)  [unwired: 1 in]
                                n235 = Number To Decimal String(number=w522) -> (decimal integer string=w531:string)  [unwired: 1 in]
                                n236 = Concatenate Strings("x" ("string"), w532, "_y" ("string"), w531, ".png" ("string")) -> (w536:string)
                                n237 = Unbundle(w527) -> ("Height"=w526:i32, "Width"=w525:i32)
                                n238 = Build Path(base path=w529, name or relative path=w536) -> (appended path=w530:path)
                                n239 = call "GetActImgMem.vi"("Camera Handle In"=w528) -> ("Image Memory Out"=w539:u8[])  [unwired: 7 in, 3 out]
                                n240 = Reshape Array(w539, w526, w525) -> (w540:u8[][])
                                n241 = call <vilib>:"Flatten Pixmap.vi"("colors"=u32[] [0, 65793, 131586, 197379, 263172, 328965, 394758, 460551, 526344, 592137, 657930, 723723, 789516, 855309, 921102, 986895, 1052688, 1118481, 1184274, 1250067, 1315860, 1381653, 1447446, 1513239, 1579032, 1644825, 1710618, 1776411, 1842204, 1907997, 1973790, 2039583, 2105376, 2171169, 2236962, 2302755, 2368548, 2434341, 2500134, 2565927, 2631720, 2697513, 2763306, 2829099, 2894892, 2960685, 3026478, 3092271, 3158064, 3223857, 3289650, 3355443, 3421236, 3487029, 3552822, 3618615, 3684408, 3750201, 3815994, 3881787, 3947580, 4013373, 4079166, 4144959, 4210752, 4276545, 4342338, 4408131, 4473924, 4539717, 4605510, 4671303, 4737096, 4802889, 4868682, 4934475, 5000268, 5066061, 5131854, 5197647, 5263440, 5329233, 5395026, 5460819, 5526612, 5592405, 5658198, 5723991, 5789784, 5855577, 5921370, 5987163, 6052956, 6118749, 6184542, 6250335, 6316128, 6381921, 6447714, 6513507, 6579300, 6645093, 6710886, 6776679, 6842472, 6908265, 6974058, 7039851, 7105644, 7171437, 7237230, 7303023, 7368816, 7434609, 7500402, 7566195, 7631988, 7697781, 7763574, 7829367, 7895160, 7960953, 8026746, 8092539, 8158332, 8224125, 8289918, 8355711, 8421504, 8487297, 8553090, 8618883, 8684676, 8750469, 8816262, 8882055, 8947848, 9013641, 9079434, 9145227, 9211020, 9276813, 9342606, 9408399, 9474192, 9539985, 9605778, 9671571, 9737364, 9803157, 9868950, 9934743, 10000536, 10066329, 10132122, 10197915, 10263708, 10329501, 10395294, 10461087, 10526880, 10592673, 10658466, 10724259, 10790052, 10855845, 10921638, 10987431, 11053224, 11119017, 11184810, 11250603, 11316396, 11382189, 11447982, 11513775, 11579568, 11645361, 11711154, 11776947, 11842740, 11908533, 11974326, 12040119, 12105912, 12171705, 12237498, 12303291, 12369084, 12434877, 12500670, 12566463, 12632256, 12698049, 12763842, 12829635, 12895428, 12961221, 13027014, 13092807, 13158600, 13224393, 13290186, 13355979, 13421772, 13487565, 13553358, 13619151, 13684944, 13750737, 13816530, 13882323, 13948116, 14013909, 14079702, 14145495, 14211288, 14277081, 14342874, 14408667, 14474460, 14540253, 14606046, 14671839, 14737632, 14803425, 14869218, 14935011, 15000804, 15066597, 15132390, 15198183, 15263976, 15329769, 15395562, 15461355, 15527148, 15592941, 15658734, 15724527, 15790320, 15856113, 15921906, 15987699, 16053492, 16119285, 16185078, 16250871, 16316664, 16382457, 16448250, 16514043, 16579836, 16645629, 16711422, 0] ("output array 2"), "8-bit pixmap"=w540) -> ("image data"=w537:T33)  [unwired: 9 in]
                                n242 = Wait (ms)(milliseconds to wait=u32 300) -> ()  [unwired: 1 out]
                                n243 = call <vilib>:"Write PNG File.vi"("image data"=w537, "path to PNG file"=w530) -> ()  [unwired: 8 in, 2 out]
                                }
                                }
                              }
                            }
                            frame True {
                              n244 = for {
                                N: w547 -> [_]
                                tunnel: w546 -> [w553]
                                tunnel: w545 -> [w552]
                                tunnel: w544 -> [w551]
                                tunnel: w543 -> [w550]
                                tunnel: w542 -> [w549]
                                tunnel: [w548] -> w541
                                i -> [w548]
                                n245 = stacked-sequence {
                                tunnel: w553 -> [_ w559 _]
                                tunnel: w552 -> [_ _ w579]
                                tunnel: w551 -> [_ _ w578]
                                tunnel: w550 -> [_ _ w576]
                                tunnel: w548 -> [_ _ w566]
                                tunnel: w549 -> [_ _ w568]
                                frame #0 {
                                n246 = Wait (ms)(milliseconds to wait=u32 100) -> ()  [unwired: 1 out]
                                }
                                frame #1 {
                                w564 = 1 items=["Forward"=1, "Backward"=2] ("direction")
                                n247 = Unbundle By Name(w559) -> ("Device X"=w558:refnum<k24>)  [unwired: 2 out]
                                n248 = Divide(x=0.0877 ("y"), y=1000.0) -> (x/y=w555:dbl)
                                n249 = Multiply(x=50.0, y=w555) -> (x*y=w560:dbl)
                                n250 = invoke class="KCubeDCServo" method="MoveRelative"(reference=w558, "direction"=w564, "stepSize"=w560, "waitTimeout"=0) -> ()  [unwired: 2 in, 6 out]
                                n251 = Wait (ms)(milliseconds to wait=u32 400) -> ()  [unwired: 1 out]
                                }
                                frame #2 {
                                n252 = Increment(x=w566) -> (x+1=w565:i32)
                                n253 = Increment(x=w568) -> (x+1=w567:i32)
                                n254 = Number To Decimal String(number=w567) -> (decimal integer string=w571:string)  [unwired: 1 in]
                                n255 = Number To Decimal String(number=w565) -> (decimal integer string=w572:string)  [unwired: 1 in]
                                n256 = Concatenate Strings("x" ("string"), w572, "_y" ("string"), w571, ".png" ("string")) -> (w577:string)
                                n257 = Build Path(base path=w576, name or relative path=w577) -> (appended path=w570:path)
                                n258 = call "GetActImgMem.vi"("Camera Handle In"=w579) -> ("Image Memory Out"=w582:u8[])  [unwired: 7 in, 3 out]
                                n259 = Unbundle(w578) -> ("Height"=w583:i32, "Width"=w584:i32)
                                n260 = Reshape Array(w582, w583, w584) -> (w585:u8[][])
                                n261 = call <vilib>:"Flatten Pixmap.vi"("colors"=u32[] [0, 65793, 131586, 197379, 263172, 328965, 394758, 460551, 526344, 592137, 657930, 723723, 789516, 855309, 921102, 986895, 1052688, 1118481, 1184274, 1250067, 1315860, 1381653, 1447446, 1513239, 1579032, 1644825, 1710618, 1776411, 1842204, 1907997, 1973790, 2039583, 2105376, 2171169, 2236962, 2302755, 2368548, 2434341, 2500134, 2565927, 2631720, 2697513, 2763306, 2829099, 2894892, 2960685, 3026478, 3092271, 3158064, 3223857, 3289650, 3355443, 3421236, 3487029, 3552822, 3618615, 3684408, 3750201, 3815994, 3881787, 3947580, 4013373, 4079166, 4144959, 4210752, 4276545, 4342338, 4408131, 4473924, 4539717, 4605510, 4671303, 4737096, 4802889, 4868682, 4934475, 5000268, 5066061, 5131854, 5197647, 5263440, 5329233, 5395026, 5460819, 5526612, 5592405, 5658198, 5723991, 5789784, 5855577, 5921370, 5987163, 6052956, 6118749, 6184542, 6250335, 6316128, 6381921, 6447714, 6513507, 6579300, 6645093, 6710886, 6776679, 6842472, 6908265, 6974058, 7039851, 7105644, 7171437, 7237230, 7303023, 7368816, 7434609, 7500402, 7566195, 7631988, 7697781, 7763574, 7829367, 7895160, 7960953, 8026746, 8092539, 8158332, 8224125, 8289918, 8355711, 8421504, 8487297, 8553090, 8618883, 8684676, 8750469, 8816262, 8882055, 8947848, 9013641, 9079434, 9145227, 9211020, 9276813, 9342606, 9408399, 9474192, 9539985, 9605778, 9671571, 9737364, 9803157, 9868950, 9934743, 10000536, 10066329, 10132122, 10197915, 10263708, 10329501, 10395294, 10461087, 10526880, 10592673, 10658466, 10724259, 10790052, 10855845, 10921638, 10987431, 11053224, 11119017, 11184810, 11250603, 11316396, 11382189, 11447982, 11513775, 11579568, 11645361, 11711154, 11776947, 11842740, 11908533, 11974326, 12040119, 12105912, 12171705, 12237498, 12303291, 12369084, 12434877, 12500670, 12566463, 12632256, 12698049, 12763842, 12829635, 12895428, 12961221, 13027014, 13092807, 13158600, 13224393, 13290186, 13355979, 13421772, 13487565, 13553358, 13619151, 13684944, 13750737, 13816530, 13882323, 13948116, 14013909, 14079702, 14145495, 14211288, 14277081, 14342874, 14408667, 14474460, 14540253, 14606046, 14671839, 14737632, 14803425, 14869218, 14935011, 15000804, 15066597, 15132390, 15198183, 15263976, 15329769, 15395562, 15461355, 15527148, 15592941, 15658734, 15724527, 15790320, 15856113, 15921906, 15987699, 16053492, 16119285, 16185078, 16250871, 16316664, 16382457, 16448250, 16514043, 16579836, 16645629, 16711422, 0] ("output array 2"), "8-bit pixmap"=w585) -> ("image data"=w580:T33)  [unwired: 9 in]
                                n262 = call <vilib>:"Write PNG File.vi"("image data"=w580, "path to PNG file"=w570) -> ()  [unwired: 8 in, 2 out]
                                n263 = Wait (ms)(milliseconds to wait=u32 300) -> ()  [unwired: 1 out]
                                }
                                }
                              }
                            }
                          }
                        }
                      }
                      n264 = Increment(x=w415) -> (x+1=→"Frame_X":i32)
                      "Total_Frame_Y" <- w416
                    }
                  }
                  frame #3 {
                    n265 = One Button Dialog(message="Scanning is finished!!!", button name ("OK")="OK") -> ()  [unwired: 1 out]
                  }
                }
              }
              event "X axis_R": Value Change {
                n266 = event-data() -> ()  [unwired: 1 in, 6 out]
                n267 = Unbundle(w597) -> ("Device X"=w595:refnum<k24>)  [unwired: 2 out]
                n268 = case shown="\"0.05mm\"" w589 {
                  tunnel: [0.01 0.1 0.5 1.0 1.5 0.05] -> w588
                  frame "0.01mm", Default {
                  }
                  frame "0.1mm" {
                  }
                  frame "0.5mm" {
                  }
                  frame "1mm" {
                  }
                  frame "1.5mm" {
                  }
                  frame "0.05mm" {
                  }
                }
                n269 = Subtract(x=12.0, y=w588) -> (x-y=w593:dbl)
                n270 = Greater?(x=w593, y=w592) -> (0:w591:bool)
                n271 = case shown="True" w591 {
                  tunnel: w595 -> [_ w610]
                  tunnel: w588 -> [_ w609]
                  frame False {
                  }
                  frame True {
                    w612 = 1 items=["Forward"=1, "Backward"=2] ("direction")
                    n272 = invoke class="KCubeDCServo" method="MoveRelative"(reference=w610, "direction"=w612, "stepSize"=w609, "waitTimeout"=0) -> ()  [unwired: 2 in, 6 out]
                  }
                }
                n273 = Wait (ms)(milliseconds to wait=u32 50) -> ()  [unwired: 1 out]
              }
              event "X axis_L": Value Change {
                n274 = event-data() -> ()  [unwired: 1 in, 6 out]
                n275 = Unbundle(w619) -> ("Device X"=w618:refnum<k24>)  [unwired: 2 out]
                n276 = case shown="\"0.05mm\"" w614 {
                  tunnel: [0.01 0.1 0.5 1.0 1.5 0.05] -> w613
                  frame "0.01mm", Default {
                  }
                  frame "0.1mm" {
                  }
                  frame "0.5mm" {
                  }
                  frame "1mm" {
                  }
                  frame "1.5mm" {
                  }
                  frame "0.05mm" {
                  }
                }
                n277 = Less?(x=w613, y=w617) -> (x < y?=w616:bool)
                n278 = case shown="True" w616 {
                  tunnel: w618 -> [_ w633]
                  tunnel: w613 -> [_ w632]
                  frame False {
                  }
                  frame True {
                    w635 = 2 items=["Forward"=1, "Backward"=2] ("direction")
                    n279 = invoke class="KCubeDCServo" method="MoveRelative"(reference=w633, "direction"=w635, "stepSize"=w632, "waitTimeout"=0) -> ()  [unwired: 2 in, 6 out]
                  }
                }
                n280 = Wait (ms)(milliseconds to wait=u32 50) -> ()  [unwired: 1 out]
              }
              event "Y axis_B": Value Change {
                n281 = event-data() -> ()  [unwired: 1 in, 6 out]
                n282 = Unbundle(w642) -> ("Device Y"=w641:refnum<k24>)  [unwired: 2 out]
                n283 = case shown="\"0.05mm\"" w637 {
                  tunnel: [0.01 0.1 0.5 1.0 1.5 0.05] -> w636
                  frame "0.01mm", Default {
                  }
                  frame "0.1mm" {
                  }
                  frame "0.5mm" {
                  }
                  frame "1mm" {
                  }
                  frame "1.5mm" {
                  }
                  frame "0.05mm" {
                  }
                }
                n284 = Subtract(x=12.0, y=w636) -> (x-y=w643:dbl)
                n285 = Greater?(x=w643, y=w639) -> (0:w640:bool)
                n286 = case shown="True" w640 {
                  tunnel: w641 -> [_ w658]
                  tunnel: w636 -> [_ w657]
                  frame False {
                  }
                  frame True {
                    w660 = 1 items=["Forward"=1, "Backward"=2] ("direction")
                    n287 = invoke class="KCubeDCServo" method="MoveRelative"(reference=w658, "direction"=w660, "stepSize"=w657, "waitTimeout"=0) -> ()  [unwired: 2 in, 6 out]
                  }
                }
                n288 = Wait (ms)(milliseconds to wait=u32 50) -> ()  [unwired: 1 out]
              }
              event "Y axis_F": Value Change {
                n289 = event-data() -> ()  [unwired: 1 in, 6 out]
                n290 = Unbundle(w666) -> ("Device Y"=w665:refnum<k24>)  [unwired: 2 out]
                n291 = case shown="\"0.05mm\"" w662 {
                  tunnel: [0.01 0.1 0.5 1.0 1.5 0.05] -> w661
                  frame "0.01mm", Default {
                  }
                  frame "0.1mm" {
                  }
                  frame "0.5mm" {
                  }
                  frame "1mm" {
                  }
                  frame "1.5mm" {
                  }
                  frame "0.05mm" {
                  }
                }
                n292 = Less?(x=w661, y=w664) -> (x < y?=w667:bool)
                n293 = case shown="True" w667 {
                  tunnel: w665 -> [_ w681]
                  tunnel: w661 -> [_ w680]
                  frame False {
                  }
                  frame True {
                    w683 = 2 items=["Forward"=1, "Backward"=2] ("direction")
                    n294 = invoke class="KCubeDCServo" method="MoveRelative"(reference=w681, "direction"=w683, "stepSize"=w680, "waitTimeout"=0) -> ()  [unwired: 2 in, 6 out]
                  }
                }
                n295 = Wait (ms)(milliseconds to wait=u32 50) -> ()  [unwired: 1 out]
              }
              event "Z axis_u": Value Change {
                n296 = event-data() -> ()  [unwired: 1 in, 6 out]
                n297 = Unbundle(w689) -> ("Device Z"=w688:refnum<k24>)  [unwired: 2 out]
                n298 = case shown="\"20step\"" w690 {
                  tunnel: [1 5 10 30 300 3000] -> w691
                  frame "1step", Default {
                  }
                  frame "2step" {
                  }
                  frame "5step" {
                  }
                  frame "10step" {
                  }
                  frame "15step" {
                  }
                  frame "20step" {
                  }
                }
                n299 = invoke class="KCubeDCServo" method="SetJogStepSize_DeviceUnit"(reference=w688, "stepSize"=w691) -> (reference out=w685:refnum<k24>)  [unwired: 2 in, 3 out]
                n300 = Less?(x=w686, y=11.5) -> (x < y?=w687:bool)
                n301 = case shown="True" w687 {
                  tunnel: w685 -> [_ w699]
                  frame False {
                  }
                  frame True {
                    w701 = 1 items=["Forward"=1, "Backward"=2] ("direction")
                    n302 = invoke class="KCubeDCServo" method="MoveJog"(reference=w699, "direction"=w701, "waitTimeout"=0) -> ()  [unwired: 2 in, 5 out]
                  }
                }
                n303 = Wait (ms)(milliseconds to wait=u32 50) -> ()  [unwired: 1 out]
              }
              event "Z axis_d": Value Change {
                n304 = event-data() -> ()  [unwired: 1 in, 6 out]
                n305 = Unbundle(w714) -> ("Device Z"=w715:refnum<k24>)  [unwired: 2 out]
                n306 = case shown="\"20step\"" w713 {
                  tunnel: [1 5 10 30 300 3000] -> w716
                  frame "1step", Default {
                  }
                  frame "2step" {
                  }
                  frame "5step" {
                  }
                  frame "10step" {
                  }
                  frame "15step" {
                  }
                  frame "20step" {
                  }
                }
                n307 = invoke class="KCubeDCServo" method="SetJogStepSize_DeviceUnit"(reference=w715, "stepSize"=w716) -> (reference out=w712:refnum<k24>)  [unwired: 2 in, 3 out]
                n308 = Less?(x=0.01 ("y"), y=w710) -> (x < y?=w711:bool)
                n309 = case shown="True" w711 {
                  tunnel: w712 -> [_ w723]
                  frame False {
                  }
                  frame True {
                    w725 = 2 items=["Forward"=1, "Backward"=2] ("direction")
                    n310 = invoke class="KCubeDCServo" method="MoveJog"(reference=w723, "direction"=w725, "waitTimeout"=0) -> ()  [unwired: 2 in, 5 out]
                  }
                }
                n311 = Wait (ms)(milliseconds to wait=u32 50) -> ()  [unwired: 1 out]
              }
              event "MoveTo": Value Change {
                n312 = event-data() -> ()  [unwired: 1 in, 6 out]
                n313 = Unbundle(w733) -> ("Device Z"=w732:refnum<k24>)  [unwired: 2 out]
                n314 = invoke class="KCubeDCServo" method="MoveTo"(reference=w732, "position"="Destination", "waitTimeout"=0) -> ()  [unwired: 2 in, 5 out]
                n315 = Wait (ms)(milliseconds to wait=u32 1000) -> ()  [unwired: 1 out]
              }
              event "ImageSnap": Value Change {
                n316 = event-data() -> ()  [unwired: 1 in, 6 out]
                n317 = call "GetActImgMem.vi"("Camera Handle In"=w752) -> ("Image Memory Out"=w747:u8[])  [unwired: 7 in, 3 out]
                n318 = Unbundle(w745) -> ("Height"=w748:i32, "Width"=w749:i32)
                n319 = Reshape Array(w747, w748, w749) -> (w750:u8[][])
                n320 = call <vilib>:"Flatten Pixmap.vi"("colors"=u32[] [0, 65793, 131586, 197379, 263172, 328965, 394758, 460551, 526344, 592137, 657930, 723723, 789516, 855309, 921102, 986895, 1052688, 1118481, 1184274, 1250067, 1315860, 1381653, 1447446, 1513239, 1579032, 1644825, 1710618, 1776411, 1842204, 1907997, 1973790, 2039583, 2105376, 2171169, 2236962, 2302755, 2368548, 2434341, 2500134, 2565927, 2631720, 2697513, 2763306, 2829099, 2894892, 2960685, 3026478, 3092271, 3158064, 3223857, 3289650, 3355443, 3421236, 3487029, 3552822, 3618615, 3684408, 3750201, 3815994, 3881787, 3947580, 4013373, 4079166, 4144959, 4210752, 4276545, 4342338, 4408131, 4473924, 4539717, 4605510, 4671303, 4737096, 4802889, 4868682, 4934475, 5000268, 5066061, 5131854, 5197647, 5263440, 5329233, 5395026, 5460819, 5526612, 5592405, 5658198, 5723991, 5789784, 5855577, 5921370, 5987163, 6052956, 6118749, 6184542, 6250335, 6316128, 6381921, 6447714, 6513507, 6579300, 6645093, 6710886, 6776679, 6842472, 6908265, 6974058, 7039851, 7105644, 7171437, 7237230, 7303023, 7368816, 7434609, 7500402, 7566195, 7631988, 7697781, 7763574, 7829367, 7895160, 7960953, 8026746, 8092539, 8158332, 8224125, 8289918, 8355711, 8421504, 8487297, 8553090, 8618883, 8684676, 8750469, 8816262, 8882055, 8947848, 9013641, 9079434, 9145227, 9211020, 9276813, 9342606, 9408399, 9474192, 9539985, 9605778, 9671571, 9737364, 9803157, 9868950, 9934743, 10000536, 10066329, 10132122, 10197915, 10263708, 10329501, 10395294, 10461087, 10526880, 10592673, 10658466, 10724259, 10790052, 10855845, 10921638, 10987431, 11053224, 11119017, 11184810, 11250603, 11316396, 11382189, 11447982, 11513775, 11579568, 11645361, 11711154, 11776947, 11842740, 11908533, 11974326, 12040119, 12105912, 12171705, 12237498, 12303291, 12369084, 12434877, 12500670, 12566463, 12632256, 12698049, 12763842, 12829635, 12895428, 12961221, 13027014, 13092807, 13158600, 13224393, 13290186, 13355979, 13421772, 13487565, 13553358, 13619151, 13684944, 13750737, 13816530, 13882323, 13948116, 14013909, 14079702, 14145495, 14211288, 14277081, 14342874, 14408667, 14474460, 14540253, 14606046, 14671839, 14737632, 14803425, 14869218, 14935011, 15000804, 15066597, 15132390, 15198183, 15263976, 15329769, 15395562, 15461355, 15527148, 15592941, 15658734, 15724527, 15790320, 15856113, 15921906, 15987699, 16053492, 16119285, 16185078, 16250871, 16316664, 16382457, 16448250, 16514043, 16579836, 16645629, 16711422, 0] ("output array 2"), "8-bit pixmap"=w750) -> ("image data"=w744:T33)  [unwired: 9 in]
                n321 = call <vilib>:"Write PNG File.vi"("image data"=w744) -> ()  [unwired: 9 in, 2 out]
              }
              event "Galvo Center": Value Change {
                n322 = event-data() -> ()  [unwired: 1 in, 6 out]
                n323 = local read "ZOffset"() -> (w771:dbl)
                n324 = local read "YOffset"() -> (w757:dbl)
                n325 = local read "XOffset"() -> (w758:dbl)
                n326 = call "aoyc"("Offset"=w757) -> ("DC"=w768:dynamicdata)  [unwired: 13 in, 1 out]
                n327 = call "aoxc"("Offset"=w758) -> ("DC"=w769:dynamicdata)  [unwired: 13 in, 1 out]
                n328 = call "aozc"("Offset"=w771) -> ("DC"=w772:dynamicdata)  [unwired: 13 in, 1 out]
                n329 = call <vilib>:"DAQmx Start Task.vi"("task/channels in"=w767, "error in"=w765) -> ("task out"=w766:refnum<k21>, "error out"=w764:errorcluster)  [unwired: 12 in]
                n330 = Build Array(w769, w768, w772) -> (w770:dynamicdata[])
                n331 = call "Galvo_Reset.vi"("error in"=w764, "auto start"=TRUE, "Signal array"=w770, "task/channels in"=w766) -> ("error out"=w761:errorcluster, "task out"=w762:refnum<k21>)  [unwired: 6 in]
                n332 = call <vilib>:"DAQmx Stop Task.vi"("task/channels in"=w762, "error in"=w761) -> ("task out"=w760:refnum<k21>, "error out"=w759:errorcluster)  [unwired: 12 in]
              }
              event "Live video": Mouse Down {
                # "When the mouse is inside the video area, after the mouse is down and hold, the coordinate of the ROI upper left corner is stored."
                n333 = event-data() -> ("Coords"=w781:T22)  [unwired: 1 in, 7 out]
              }
              event "Live video": Mouse Up {
                # "When the mouse is inside the video area, after the mouse is up, the edge of the ROI is calculated."
                n334 = event-data() -> ("Coords"=w790:T22)  [unwired: 1 in, 7 out]
                n335 = property on="Live video" class="Pict"() -> ("Position"=w788:T34)  [unwired: 2 in, 2 out]
                n336 = Unbundle By Name "Start"(w789) -> ("Horizontal"=w810:i32, "Vertical"=w807:i32)
                n337 = Unbundle By Name(w790) -> ("Horizontal"=w804:i32, "Vertical"=w801:i32)
                n338 = Unbundle By Name(w788) -> ("Left"=w812:i32, "Top"=w811:i32)
                n339 = Subtract(x=w810, y=3) -> (x-y=w808:i32)
                n340 = Subtract(x=w807, y=3) -> (x-y=w806:i32)
                n341 = Subtract(x=w804, y=3) -> (x-y=w802:i32)
                n342 = Subtract(x=w801, y=3) -> (x-y=w799:i32)
                n343 = Subtract(x=w808, y=w812) -> (x-y=w798:i32)
                n344 = Subtract(x=w806, y=w811) -> (x-y=w797:i32)
                n345 = Subtract(x=w802, y=w812) -> (x-y=w784:i32)
                n346 = Subtract(x=w799, y=w811) -> (x-y=w783:i32)
                n347 = Divide(x=w798, y=w791) -> (x/y=w796:dbl)
                n348 = Divide(x=w797, y=w791) -> (x/y=w795:dbl)
                n349 = Divide(x=w784, y=w791) -> (x/y=w794:dbl)
                n350 = Divide(x=w783, y=w791) -> (x/y=w793:dbl)
                n351 = Bundle By Name(cluster=T21 {"left"=0, "top"=0, "right"=0, "bottom"=0} ("rect"), "left"=w796, "top"=w795, "right"=w794, "bottom"=w793) -> (w792:T21)
              }
              event "Quit": Value Change {
                # "Add recover initial position\nZ: max\nX: middle\nY: middle\nand also need to attch a limit"
                # "When user clicks the STOP button, program will jump to \"Shut down\" state"
                n352 = event-data() -> ()  [unwired: 1 in, 6 out]
              }
              event "Focus": Value Change {
                # "When clicking the Focus button, following steps will be executed: \n1. move the stage to 4 different Z positions and take an image at each position;\n2. crop the image to get 4 ROIs and use them to find the focal plane;\n3. move the stage to the focal plane."
                n353 = event-data() -> ()  [unwired: 1 in, 6 out]
                n354 = Divide(x="Jog size (um)", y=1000.0) -> (x/y=w823:dbl)
                n355 = Divide(x=w823, y=2.0) -> (x/y=w825:dbl)
                n356 = call "StageReadPos.vi"("error in (no error)"=w866, "Stage Select"=StageSelect."Z axis", "Device In"=w837) -> ("error out"=w864:errorcluster, "CurrentPosition"=w830:dbl)  [unwired: 7 in]
                n357 = Unbundle By Name(w859) -> ("Device Z"=w856:refnum<k24>)
                n358 = Add(x=w830, y=w823) -> (x+y=w828:dbl)
                n359 = Subtract(x=w830, y=w823) -> (x-y=w860:dbl)
                n360 = invoke class="KCubeDCServo" method="GetVelocityParams"(reference=w856) -> ("GetVelocityParams"=w855:refnum<k24>)  [unwired: 2 in, 2 out]
                n361 = Subtract(x=w830, y=w825) -> (x-y=w831:dbl)
                n362 = Subtract(x=w828, y=w825) -> (x-y=w829:dbl)
                n363 = Add(x=w829, y=w823) -> (x+y=w826:dbl)
                n364 = Subtract(x=w860, y=w825) -> (x-y=w824:dbl)
                n365 = Subtract(x=w826, y=w825) -> (x-y=w827:dbl)
                n366 = Build Array(w824, w831, w829, w827) -> (w857:dbl[])
                n367 = property class="VelocityParameters"(reference=w855) -> (reference out=w853:refnum<k24>, error out=w854:errorcluster, "Acceleration"=w852:dbl)  [unwired: 1 in]
                n368 = property class="VelocityParameters"(reference=w853, error in=w854) -> ("MaxVelocity"=w851:dbl)  [unwired: 2 out]
                n369 = for {
                  tunnel: w857 -> [w895] mode=indexing
                  tunnel: w864 -> [w898]
                  tunnel: w837 -> [w897]
                  tunnel: [w888] -> w858
                  tunnel: w863 -> [w891]
                  tunnel: w862 -> [w890]
                  tunnel: [w870] -> w846 mode=indexing
                  tunnel: w861 -> [w886]
                  tunnel: w823 -> [w884]
                  tunnel: w852 -> [w875]
                  tunnel: w851 -> [w874]
                  w878 = 0.9 ("y")
                  n370 = call "StageToPos.vi"("error in (no error)"=w898, "Move to pos"=w895, "Stage Select"=StageSelect."Z axis", "Device In"=w897) -> ("error out"=w883:errorcluster)  [unwired: 7 in]
                  n371 = call "MovingTime.vi"("error in"=w883, "Acc (mm/s^2)"=w875, "MaxV (mm/s)"=w874, "Distance (mm)"=w884) -> ("error out"=w882:errorcluster, "time (s)"=w881:dbl)  [unwired: 6 in]
                  n372 = Multiply(x=w881, y=2.0) -> (x*y=w877:dbl)
                  n373 = Greater?(x=w877, y=w878) -> (0:w879:bool)
                  n374 = Select(t=w877, s=w879, f=w878) -> (s? t:f=w876:dbl)
                  "Delay (s)" <- w876
                  n375 = call "Time Delay"("error in (no error)"=w882, "Delay Time (s)"=w876) -> ("error out"=w885:errorcluster)  [unwired: 9 in]
                  n376 = call "GetActImgMem.vi"("error in"=w885, "Camera Handle In"=w891) -> ("error out"=w889:errorcluster, "Image Memory Out"=w892:u8[])  [unwired: 6 in, 2 out]
                  n377 = Unbundle(w890) -> ("Height"=w893:i32, "Width"=w894:i32)
                  n378 = Reshape Array(w892, w893, w894) -> (w869:u8[][])
                  n379 = call <vilib>:"Flatten Pixmap.vi"("colors"=u32[] [0, 65793, 131586, 197379, 263172, 328965, 394758, 460551, 526344, 592137, 657930, 723723, 789516, 855309, 921102, 986895, 1052688, 1118481, 1184274, 1250067, 1315860, 1381653, 1447446, 1513239, 1579032, 1644825, 1710618, 1776411, 1842204, 1907997, 1973790, 2039583, 2105376, 2171169, 2236962, 2302755, 2368548, 2434341, 2500134, 2565927, 2631720, 2697513, 2763306, 2829099, 2894892, 2960685, 3026478, 3092271, 3158064, 3223857, 3289650, 3355443, 3421236, 3487029, 3552822, 3618615, 3684408, 3750201, 3815994, 3881787, 3947580, 4013373, 4079166, 4144959, 4210752, 4276545, 4342338, 4408131, 4473924, 4539717, 4605510, 4671303, 4737096, 4802889, 4868682, 4934475, 5000268, 5066061, 5131854, 5197647, 5263440, 5329233, 5395026, 5460819, 5526612, 5592405, 5658198, 5723991, 5789784, 5855577, 5921370, 5987163, 6052956, 6118749, 6184542, 6250335, 6316128, 6381921, 6447714, 6513507, 6579300, 6645093, 6710886, 6776679, 6842472, 6908265, 6974058, 7039851, 7105644, 7171437, 7237230, 7303023, 7368816, 7434609, 7500402, 7566195, 7631988, 7697781, 7763574, 7829367, 7895160, 7960953, 8026746, 8092539, 8158332, 8224125, 8289918, 8355711, 8421504, 8487297, 8553090, 8618883, 8684676, 8750469, 8816262, 8882055, 8947848, 9013641, 9079434, 9145227, 9211020, 9276813, 9342606, 9408399, 9474192, 9539985, 9605778, 9671571, 9737364, 9803157, 9868950, 9934743, 10000536, 10066329, 10132122, 10197915, 10263708, 10329501, 10395294, 10461087, 10526880, 10592673, 10658466, 10724259, 10790052, 10855845, 10921638, 10987431, 11053224, 11119017, 11184810, 11250603, 11316396, 11382189, 11447982, 11513775, 11579568, 11645361, 11711154, 11776947, 11842740, 11908533, 11974326, 12040119, 12105912, 12171705, 12237498, 12303291, 12369084, 12434877, 12500670, 12566463, 12632256, 12698049, 12763842, 12829635, 12895428, 12961221, 13027014, 13092807, 13158600, 13224393, 13290186, 13355979, 13421772, 13487565, 13553358, 13619151, 13684944, 13750737, 13816530, 13882323, 13948116, 14013909, 14079702, 14145495, 14211288, 14277081, 14342874, 14408667, 14474460, 14540253, 14606046, 14671839, 14737632, 14803425, 14869218, 14935011, 15000804, 15066597, 15132390, 15198183, 15263976, 15329769, 15395562, 15461355, 15527148, 15592941, 15658734, 15724527, 15790320, 15856113, 15921906, 15987699, 16053492, 16119285, 16185078, 16250871, 16316664, 16382457, 16448250, 16514043, 16579836, 16645629, 16711422, 0] ("output array 2"), "8-bit pixmap"=w869) -> ("image data"=w873:T33)  [unwired: 9 in]
                  n380 = call <vilib>:"Draw Flattened Pixmap.vi"("image data"=w873) -> ("new picture"=w871:picture)  [unwired: 8 in]
                  n381 = local write "Live video"(w871) -> ()
                  n382 = call "ROI_crop.vi"("error constant"=w889, "roiEdge"=w886, "InputImage"=w869) -> ("error constant 2"=w888:errorcluster, "ROI"=w887:dbl[][])  [unwired: 7 in]
                  n383 = To Unsigned Byte Integer(number=w887) -> (unsigned 8bit integer=w870:u8[][])
                }
                n384 = Index Array(array=w846, index (dim 0)=0 ("index (page)")) -> (element=w844:u8[][])  [unwired: 2 in]
                n385 = Index Array(array=w846, index (dim 0)=1 ("index (page)")) -> (element=w843:u8[][])  [unwired: 2 in]
                n386 = Index Array(array=w846, index (dim 0)=2 ("index (page)")) -> (element=w842:u8[][])  [unwired: 2 in]
                n387 = Index Array(array=w846, index (dim 0)=3 ("index (page)")) -> (element=w841:u8[][])  [unwired: 2 in]
                n388 = Bundle By Name(cluster=T29 {"Image2"=[], "Image3"=[], "Image4"=[], "Image1"=[]} ("Imput images"), "Image1"=w844, "Image2"=w843, "Image3"=w842, "Image4"=w841) -> (w840:T29)
                n389 = call "Find_Focus.vi"("error in (no error)"=w858, "Input_Z"=w857, "Imput images"=w840) -> ("error out"=w839:errorcluster, "BestPosition"=w835:dbl)  [unwired: 7 in]
                "Focal plane (mm)" <- w835
                n390 = call "StageToPos.vi"("error in (no error)"=w839, "Move to pos"=w835, "Stage Select"=StageSelect."Z axis", "Device In"=w837) -> ("error out"=w838:errorcluster)  [unwired: 7 in]
              }
              event "Aim": Value Change {
                # "First, you need to draw an ROI, and then when you click the Aim button, the center of the\nview will move to the center of the selected ROI."
                n391 = event-data() -> ()  [unwired: 1 in, 6 out]
                n392 = Unbundle By Name(w935) -> ("left"=w933:i16, "right"=w934:i16, "top"=w928:i16, "bottom"=w927:i16)
                n393 = Unbundle By Name(w901) -> ("Laser X"=w900:dbl, "Laser Y"=w899:dbl)
                n394 = Add(x=w933, y=w934) -> (x+y=w932:i16)
                n395 = Add(x=w928, y=w927) -> (x+y=w929:i16)
                n396 = Divide(x=w932, y=i16 2) -> (x/y=w926:dbl)
                n397 = Divide(x=w929, y=i16 2) -> (x/y=w925:dbl)
                n398 = Subtract(x=w926, y=w900) -> (x-y=w915:dbl)
                n399 = Subtract(x=w925, y=w899) -> (x-y=w920:dbl)
                n400 = Divide(x="Pixel Size Y (um)", y=1000.0) -> (x/y=w916:dbl)
                n401 = Divide(x="Pixel Size X (um)", y=1000.0) -> (x/y=w914:dbl)
                n402 = Multiply(x=w914, y=w915) -> (x*y=w921:dbl)
                n403 = Multiply(x=w920, y=w916) -> (x*y=w919:dbl)
                n404 = call "StageReadPos.vi"("error in (no error)"=w936, "Stage Select"=StageSelect."X axis", "Device In"=w924) -> ("error out"=w913:errorcluster, "CurrentPosition"=w910:dbl)  [unwired: 7 in]
                n405 = call "StageReadPos.vi"("error in (no error)"=w936, "Stage Select"=StageSelect."Y axis", "Device In"=w924) -> ("error out"=w906:errorcluster, "CurrentPosition"=w905:dbl)  [unwired: 7 in]
                n406 = Add(x=w919, y=w905) -> (x+y=w904:dbl)
                n407 = Add(x=w921, y=w910) -> (x+y=w909:dbl)
                n408 = call "StageToPos.vi"("error in (no error)"=w913, "Move to pos"=w909, "Stage Select"=StageSelect."X axis", "Device In"=w924) -> ("error out"=w903:errorcluster)  [unwired: 7 in]
                n409 = call "StageToPos.vi"("error in (no error)"=w906, "Move to pos"=w904, "Stage Select"=StageSelect."Y axis", "Device In"=w924) -> ("error out"=w902:errorcluster)  [unwired: 7 in]
                n410 = Merge Errors(w903, w902) -> (w937:errorcluster)
              }
              event "LaserSpot": Value Change {
                # "First, you need to draw an ROI, and then when you click the Here's Laser button, the center of the\nROI will be stored for Aim use."
                n411 = event-data() -> ()  [unwired: 1 in, 6 out]
                n412 = Unbundle By Name(w946) -> ("left"=w953:i16, "right"=w954:i16, "top"=w948:i16, "bottom"=w947:i16)
                n413 = Add(x=w953, y=w954) -> (x+y=w952:i16)
                n414 = Add(x=w948, y=w947) -> (x+y=w949:i16)
                n415 = Divide(x=w952, y=i16 2) -> (x/y=w942:dbl)
                n416 = Divide(x=w949, y=i16 2) -> (x/y=w941:dbl)
                n417 = Bundle By Name(cluster=T20 {"Laser X"=0.0, "Laser Y"=0.0} ("LaserSpot"), "Laser X"=w942, "Laser Y"=w941) -> (w944:T20)
                n418 = local write "Spot X"(w942) -> ()
                n419 = local write "Spot Y"(w941) -> ()
                "Boolean" <- TRUE ("Boolean")
              }
              event "Left": Value Change {
                n420 = event-data() -> ()  [unwired: 1 in, 6 out]
                n421 = Unbundle By Name(w962) -> ("Laser X"=w960:dbl, "Laser Y"=w961:dbl)
                n422 = Decrement(x=w960) -> (x-1=w959:dbl)
                n423 = Bundle By Name(cluster=T20 {"Laser X"=0.0, "Laser Y"=0.0} ("LaserSpot"), "Laser X"=w959, "Laser Y"=w961) -> (w963:T20)
                n424 = local write "Spot X"(w959) -> ()
              }
              event "Right": Value Change {
                n425 = event-data() -> ()  [unwired: 1 in, 6 out]
                n426 = Unbundle By Name(w973) -> ("Laser X"=w971:dbl, "Laser Y"=w974:dbl)
                n427 = Increment(x=w971) -> (x+1=w970:dbl)
                n428 = Bundle By Name(cluster=T20 {"Laser X"=0.0, "Laser Y"=0.0} ("LaserSpot"), "Laser X"=w970, "Laser Y"=w974) -> (w972:T20)
                n429 = local write "Spot X"(w970) -> ()
              }
              event "Up": Value Change {
                n430 = event-data() -> ()  [unwired: 1 in, 6 out]
                n431 = Unbundle By Name(w985) -> ("Laser X"=w983:dbl, "Laser Y"=w982:dbl)
                n432 = Decrement(x=w982) -> (x-1=w981:dbl)
                n433 = Bundle By Name(cluster=T20 {"Laser X"=0.0, "Laser Y"=0.0} ("LaserSpot"), "Laser X"=w983, "Laser Y"=w981) -> (w984:T20)
                n434 = local write "Spot Y"(w981) -> ()
              }
              event "Down": Value Change {
                n435 = event-data() -> ()  [unwired: 1 in, 6 out]
                n436 = Unbundle By Name(w996) -> ("Laser X"=w994:dbl, "Laser Y"=w993:dbl)
                n437 = Increment(x=w993) -> (x+1=w992:dbl)
                n438 = Bundle By Name(cluster=T20 {"Laser X"=0.0, "Laser Y"=0.0} ("LaserSpot"), "Laser X"=w994, "Laser Y"=w992) -> (w995:T20)
                n439 = local write "Spot Y"(w992) -> ()
              }
              event "Galvo Scan": Value Change {
                w1033 = 2.0 ("y")
                w1062 = 2
                w1063 = T26."Disabled and Grayed Out" ("Disabled")
                n440 = event-data() -> ()  [unwired: 1 in, 6 out]
                n441 = local read "Scan Resolusion"() -> (w1049:T2)
                n442 = local read "Box"() -> (w1052:cluster{"Width":dbl, " Height":dbl})
                n443 = local read "Scan Range"() -> (w1046:T1)
                n444 = Unbundle By Name(w1046) -> ("Ver_V/H"=w1019:dbl, "Hor_V/W"=w1018:dbl, "Ver_r"=w1044:dbl, "Hor_r"=w1042:dbl)
                n445 = Unbundle By Name(w1049) -> ("Ver_V"=w1047:dbl, "Hor_H"=w1020:dbl, "Ver_Pix"=w1048:dbl, "Hor_Pix"=w1021:dbl)
                n446 = call <vilib>:"DAQmx Start Task.vi"("task/channels in"=w1066, "error in"=w1004) -> ("task out"=w1038:refnum<k21>, "error out"=w1040:errorcluster)  [unwired: 12 in]
                n447 = Unbundle By Name(w1008) -> ("Laser X"=w1059:dbl, "Laser Y"=w1058:dbl)
                n448 = Unbundle By Name(w1052) -> ("Width"=w1051:dbl, "Height"=w1050:dbl)
                n449 = Divide(x=w1021, y=w1020) -> (x/y=w1024:dbl)
                n450 = Divide(x=w1048, y=w1047) -> (x/y=w1025:dbl)
                n451 = Multiply(x=w1025, y=w1019) -> (x*y=w1045:dbl)
                n452 = Multiply(x=w1024, y=w1018) -> (x*y=w1043:dbl)
                n453 = Get Date/Time In Seconds() -> (seconds since 1Jan1904=w1011:timestamp)
                n454 = Divide(x=w1045, y=w1044) -> (x/y=w1041:dbl)
                n455 = Divide(x=w1051, y=w1062) -> (x/y=w1057:dbl)
                n456 = Subtract(x=w1059, y=w1057) -> (x-y=w1055:dbl)
                n457 = Divide(x=w1050, y=w1062) -> (x/y=w1056:dbl)
                n458 = Divide(x=w1043, y=w1042) -> (x/y=w1022:dbl)
                n459 = Subtract(x=w1058, y=w1056) -> (x-y=w1054:dbl)
                n460 = Round To Nearest(number=w1041) -> (nearest integer value=w1017:dbl)
                n461 = Format Date/Time String(time format string (%c)="%Y%m%d%H%M%S", seconds (now)=w1011) -> (date/time string=w1009:string)  [unwired: 1 in]
                n462 = Add(x=w1056, y=w1058) -> (x+y=w1060:dbl)
                n463 = Add(x=w1059, y=w1057) -> (x+y=w1061:dbl)
                n464 = Divide(x=w1018, y=w1033) -> (x/y=w1029:dbl)
                n465 = Decrement(x=w1017) -> (x-1=w1016:dbl)
                n466 = local read "XOffset"() -> (w1032:dbl)
                n467 = local read "YOffset"() -> (w1030:dbl)
                n468 = local read "ZOffset"() -> (w1026:dbl)
                n469 = Divide(x=w1019, y=w1033) -> (x/y=w1031:dbl)
                n470 = Round To Nearest(number=w1022) -> (nearest integer value=w1015:dbl)
                n471 = Divide(x=w1019, y=w1016) -> (x/y=w1013:dbl)
                n472 = Bundle By Name(cluster=T21 {"left"=0, "top"=0, "right"=0, "bottom"=0} ("rect"), "left"=w1055, "top"=w1054, "right"=w1061, "bottom"=w1060) -> (w1005:T21)
                n473 = Decrement(x=w1015) -> (x-1=w1014:dbl)
                n474 = Divide(x=w1018, y=w1014) -> (x/y=w1012:dbl)
                n475 = Subtract(x=w1032, y=w1031) -> (x-y=w1028:dbl)
                n476 = Add(x=w1030, y=w1029) -> (x+y=w1027:dbl)
                n477 = property on="Galvo Scan" class="Bool"("DisabledEnum"=w1063) -> ()  [unwired: 2 in, 2 out]
                n478 = property on="Galvo Center" class="Bool"("DisabledEnum"=w1063) -> ()  [unwired: 2 in, 2 out]
                n479 = for {
                  N: w1017 -> [_]
                  tunnel: [FALSE ("Galvo")] -> w1039
                  shift-right: [w1086] -> w1036
                  shift-left: w1040 -> [w1085]
                  shift-right: [w1079] -> _
                  shift-left: w1028 -> [w1080]
                  shift-right: [w1083] -> w1037
                  shift-left: w1038 -> [w1084]
                  tunnel: w1027 -> [w1082]
                  tunnel: w1026 -> [w1081]
                  shift-right: [w1077] -> _
                  shift-left: 1 -> [w1078]
                  tunnel: w1015 -> [w1076]
                  tunnel: w1013 -> [w1075]
                  tunnel: w1012 -> [w1074]
                  tunnel: w1009 -> [w1073]
                  tunnel: w1008 -> [w1072]
                  tunnel: w1007 -> [w1071]
                  tunnel: w1006 -> [w1070]
                  tunnel: w1005 -> [w1069]
                  tunnel: w1004 -> [w1068]
                  n480 = for {
                    N: w1076 -> [_]
                    shift-right: [w1106] -> w1086
                    shift-left: w1085 -> [w1111]
                    shift-right: [w1100] -> _
                    shift-left: w1082 -> [w1102]
                    shift-right: [w1099] -> _
                    shift-left: w1081 -> [w1101]
                    shift-right: [w1104] -> w1083
                    shift-left: w1084 -> [w1105]
                    tunnel: w1080 -> [w1103]
                    tunnel: [w1098] -> w1079
                    shift-right: [w1088] -> w1077
                    shift-left: w1078 -> [w1097]
                    tunnel: w1075 -> [w1096]
                    tunnel: w1074 -> [w1095]
                    tunnel: w1073 -> [w1094]
                    tunnel: w1072 -> [w1093]
                    tunnel: w1071 -> [w1092]
                    tunnel: w1070 -> [w1091]
                    tunnel: w1069 -> [w1090]
                    tunnel: w1068 -> [w1089]
                    n481 = feedback #1() -> (w1109:errorcluster)  [unwired: 1 in]
                    n482 = feedback #2() -> (w1107:errorcluster)  [unwired: 1 in]
                    n483 = stacked-sequence {
                      tunnel: w1111 -> [w1118 _ _ _]
                      tunnel: [w1117 _ _ _] -> w1110
                      tunnel: w1109 -> [_ _ w1176 _]
                      tunnel: [_ _ w1177 _] -> w1108
                      tunnel: w1107 -> [_ _ _ w1209]
                      tunnel: [_ _ _ w1209] -> w1106
                      tunnel: w1105 -> [w1122 _ _ _]
                      tunnel: [w1121 _ _ _] -> w1104
                      tunnel: w1103 -> [w1120 _ _ _]
                      tunnel: w1102 -> [w1119 _ _ _]
                      tunnel: w1101 -> [w1115 _ _ _]
                      tunnel: [w1116 _ _ _] -> w1100
                      tunnel: [w1115 _ _ _] -> w1099
                      tunnel: [w1114 _ _ _] -> w1098
                      tunnel: w1097 -> [_ _ w1174 _]
                      tunnel: w1096 -> [w1113 _ _ _]
                      tunnel: w1095 -> [w1112 _ _ _]
                      tunnel: w1094 -> [_ _ w1171 _]
                      tunnel: w1093 -> [_ w1133 _ _]
                      tunnel: w1092 -> [_ w1132 _ _]
                      tunnel: w1091 -> [_ w1131 _ _]
                      tunnel: w1090 -> [_ w1130 _ _]
                      tunnel: w1089 -> [_ w1129 _ _]
                      tunnel: [_ _ w1172 _] -> w1088
                      frame #0 {
                        w1125 = FALSE ("SaveStatus")
                        # "move galvo"
                        n484 = Add(x=w1120, y=w1113) -> (x+y=w1114:dbl)
                        n485 = Subtract(x=w1119, y=w1112) -> (x-y=w1116:dbl)
                        n486 = call "aoy10"("Offset"=w1116) -> ("DC"=w1126:dynamicdata)  [unwired: 13 in, 1 out]
                        n487 = call "aox10"("Offset"=w1114) -> ("DC"=w1127:dynamicdata)  [unwired: 13 in, 1 out]
                        n488 = call "aoz10"("Offset"=w1115) -> ("DC"=w1128:dynamicdata)  [unwired: 13 in, 1 out]
                        n489 = Build Array(w1127, w1126, w1128) -> (w1123:dynamicdata[])
                        n490 = local write "SaveStatus"(w1125) -> ()
                        n491 = local write "Andor"(w1125) -> ()
                        n492 = call "Galvo_Reset.vi"("error in"=w1118, "auto start"=TRUE, "Signal array"=w1123, "task/channels in"=w1122) -> ("error out"=w1117:errorcluster, "task out"=w1121:refnum<k21>)  [unwired: 6 in]
                      }
                      frame #1 {
                        n493 = stacked-sequence {
                          tunnel: w1131 -> [_ w1140]
                          tunnel: w1130 -> [_ w1139]
                          tunnel: w1133 -> [_ w1138]
                          tunnel: w1132 -> [_ w1137]
                          tunnel: w1129 -> [_ w1136]
                          frame #0 {
                            "Galvo" <- TRUE
                          }
                          frame #1 {
                            n494 = stacked-sequence {
                              seq-local: [w1144 _] -> [_ w1160]
                              seq-local: [w1142 _] -> [_ w1151]
                              tunnel: w1140 -> [w1143 _]
                              tunnel: w1137 -> [w1142 _]
                              tunnel: w1136 -> [w1141 _]
                              tunnel: [_ w1156] -> w1135
                              tunnel: w1139 -> [_ w1153]
                              tunnel: w1138 -> [_ w1152]
                              frame #0 {
                                n495 = call "GetActImgMem.vi"("error in"=w1141, "Camera Handle In"=w1143) -> ("Image Memory Out"=w1144:u8[])  [unwired: 6 in, 3 out]
                              }
                              frame #1 {
                                # "Display Image"
                                n496 = Unbundle(w1151) -> ("Height"=w1150:i32, "Width"=w1149:i32)
                                n497 = Reshape Array(w1160, w1150, w1149) -> (w1159:u8[][])
                                n498 = call <vilib>:"Flatten Pixmap.vi"("colors"=u32[] [0, 65793, 131586, 197379, 263172, 328965, 394758, 460551, 526344, 592137, 657930, 723723, 789516, 855309, 921102, 986895, 1052688, 1118481, 1184274, 1250067, 1315860, 1381653, 1447446, 1513239, 1579032, 1644825, 1710618, 1776411, 1842204, 1907997, 1973790, 2039583, 2105376, 2171169, 2236962, 2302755, 2368548, 2434341, 2500134, 2565927, 2631720, 2697513, 2763306, 2829099, 2894892, 2960685, 3026478, 3092271, 3158064, 3223857, 3289650, 3355443, 3421236, 3487029, 3552822, 3618615, 3684408, 3750201, 3815994, 3881787, 3947580, 4013373, 4079166, 4144959, 4210752, 4276545, 4342338, 4408131, 4473924, 4539717, 4605510, 4671303, 4737096, 4802889, 4868682, 4934475, 5000268, 5066061, 5131854, 5197647, 5263440, 5329233, 5395026, 5460819, 5526612, 5592405, 5658198, 5723991, 5789784, 5855577, 5921370, 5987163, 6052956, 6118749, 6184542, 6250335, 6316128, 6381921, 6447714, 6513507, 6579300, 6645093, 6710886, 6776679, 6842472, 6908265, 6974058, 7039851, 7105644, 7171437, 7237230, 7303023, 7368816, 7434609, 7500402, 7566195, 7631988, 7697781, 7763574, 7829367, 7895160, 7960953, 8026746, 8092539, 8158332, 8224125, 8289918, 8355711, 8421504, 8487297, 8553090, 8618883, 8684676, 8750469, 8816262, 8882055, 8947848, 9013641, 9079434, 9145227, 9211020, 9276813, 9342606, 9408399, 9474192, 9539985, 9605778, 9671571, 9737364, 9803157, 9868950, 9934743, 10000536, 10066329, 10132122, 10197915, 10263708, 10329501, 10395294, 10461087, 10526880, 10592673, 10658466, 10724259, 10790052, 10855845, 10921638, 10987431, 11053224, 11119017, 11184810, 11250603, 11316396, 11382189, 11447982, 11513775, 11579568, 11645361, 11711154, 11776947, 11842740, 11908533, 11974326, 12040119, 12105912, 12171705, 12237498, 12303291, 12369084, 12434877, 12500670, 12566463, 12632256, 12698049, 12763842, 12829635, 12895428, 12961221, 13027014, 13092807, 13158600, 13224393, 13290186, 13355979, 13421772, 13487565, 13553358, 13619151, 13684944, 13750737, 13816530, 13882323, 13948116, 14013909, 14079702, 14145495, 14211288, 14277081, 14342874, 14408667, 14474460, 14540253, 14606046, 14671839, 14737632, 14803425, 14869218, 14935011, 15000804, 15066597, 15132390, 15198183, 15263976, 15329769, 15395562, 15461355, 15527148, 15592941, 15658734, 15724527, 15790320, 15856113, 15921906, 15987699, 16053492, 16119285, 16185078, 16250871, 16316664, 16382457, 16448250, 16514043, 16579836, 16645629, 16711422, 0] ("output array 2"), "8-bit pixmap"=w1159) -> ("image data"=w1158:T33)  [unwired: 9 in]
                                n499 = call <vilib>:"Draw Flattened Pixmap.vi"("image data"=w1158) -> ("new picture"=w1147:picture)  [unwired: 8 in]
                                n500 = case shown="True" TRUE {
                                tunnel: w1147 -> [w1161 w1167]
                                tunnel: [w1161 w1168] -> w1148
                                tunnel: w1153 -> [_ w1164]
                                tunnel: w1152 -> [_ w1163]
                                frame False {
                                }
                                frame True {
                                n501 = call <vilib>:"Draw Rectangle.vi"("picture"=w1167, "rect"=w1164, "color(black)"=u32 6618880) -> ("new picture"=w1166:picture)  [unwired: 6 in]
                                n502 = To Word Integer(number=w1163) -> (16bit integer=w1162:cluster{"Laser X":i16, "Laser Y":i16})
                                n503 = call <vilib>:"Draw Point.vi"("picture"=w1166, "point(x,y)"=w1162, "color(black)"=u32 16711680, "pen"=T27 {"Width"=5, "Style"=enum."Solid"}) -> ("new picture"=w1168:picture)  [unwired: 5 in]
                                }
                                }
                                n504 = local write "Live video"(w1148) -> ()
                                n505 = local read "Frame rate"() -> (w1146:dbl)
                                n506 = Reciprocal(x=w1146) -> (1/x=w1155:dbl)
                                n507 = Multiply(x=w1155, y=1000) -> (x*y=w1156:dbl)
                              }
                            }
                            n508 = Wait Until Next ms Multiple(millisecond multiple=w1135) -> ()  [unwired: 1 out]
                          }
                        }
                      }
                      frame #2 {
                        n509 = flat-sequence {
                          tunnel: w1176 -> [w1183]
                          tunnel: [w1182] -> w1175
                          tunnel: w1174 -> [w1180]
                          tunnel: [w1179] -> w1173
                          tunnel: w1171 -> [w1178]
                          tunnel: [w1198] -> w1177
                          tunnel: w1175 -> [w1197]
                          tunnel: w1173 -> [w1196]
                          tunnel: [w1196] -> w1172
                          frame #0 {
                            n510 = case shown="No Error" w1183 {
                              tunnel: [w1191 w1195] -> w1182
                              tunnel: [w1190 w1193] -> w1179
                              tunnel: w1183 -> [w1189 w1195]
                              tunnel: [w1188 FALSE ("SaveStatus")] -> w1181
                              tunnel: w1180 -> [w1187 w1193]
                              tunnel: w1178 -> [w1186 _]
                              frame No Error {
                                n511 = local read "FilePath"() -> (w1192:string)
                                n512 = local read "AcqSet"() -> (w1185:T11)
                                n513 = Unbundle By Name(w1185) -> ("KineticNum"=w1184:i32)
                                n514 = call "AndorSaveasSif_Ver2.vi"("Time"=w1186, "error in"=w1189, "No."=w1187, "KinNumber"=w1184, "FilePath"=w1192) -> ("error out"=w1191:errorcluster, "SaveStatus"=w1188:bool)  [unwired: 5 in]
                                n515 = Increment(x=w1187) -> (x+1=w1190:i32)
                                "CurrentFrame" <- w1187
                              }
                              frame Error {
                              }
                            }
                            n516 = local write "SaveStatus"(w1181) -> ()
                          }
                          frame #1 {
                            n517 = flat-sequence {
                              tunnel: [w1203] -> w1200
                              tunnel: [TRUE] -> w1199
                              tunnel: w1197 -> [w1201]
                              frame #0 {
                                n518 = call <userlib>:"StartAcquisition.vi"("error in (no error)"=w1201) -> ("error out"=w1203:errorcluster)  [unwired: 1 in, 1 out]
                              }
                            }
                            n519 = local write "Andor"(w1199) -> ()
                            n520 = while {
                              tunnel: w1200 -> [w1208]
                              tunnel: [w1204] -> w1198
                              stop <- w1205 continue-if-true
                              n521 = call <userlib>:"GetStatus.vi"("error in (no error)"=w1208) -> ("error out"=w1204:errorcluster, "status"=w1207:T30)  [unwired: 2 in, 1 out]
                              n522 = Equal?(x=w1207, y=Error_Code_Enum_typedef."DRV_ACQUIRING") -> (x = y?=w1205:bool)
                              "Andor" <- w1205
                            }
                          }
                        }
                      }
                      frame #3 {
                        n523 = local write "Galvo"(FALSE ("Galvo")) -> ()
                      }
                    }
                    n524 = feedback-in #1(w1110) -> ()
                    n525 = feedback-in #2(w1108) -> ()
                  }
                }
                n526 = property on="Galvo Stop" class="Bool"("DisabledEnum"=T26."Enabled" ("Disabled")) -> ()  [unwired: 2 in, 2 out]
                n527 = local write "Galvo"(w1039) -> ()
                n528 = call <vilib>:"DAQmx Stop Task.vi"("task/channels in"=w1037, "error in"=w1036) -> ("task out"=w1034:refnum<k21>, "error out"=w1035:errorcluster)  [unwired: 12 in]
              }
              event "Galvo Stop": Value Change {
                w1212 = T26."Enabled" ("Disabled")
                n529 = event-data() -> ()  [unwired: 1 in, 6 out]
                n530 = property on="Galvo Scan" class="Bool"("DisabledEnum"=w1212) -> ()  [unwired: 2 in, 2 out]
                n531 = property on="Galvo Center" class="Bool"("DisabledEnum"=w1212) -> ()  [unwired: 2 in, 2 out]
              }
            }
          }
        }
      }
      n532 = call <vilib>:"Simple Error Handler.vi"("error in (no error)"=w10) -> ()  [unwired: 4 in, 5 out]
    }
  }
  n533 = while {
    stop <- w1218 stop-if-true
    n534 = local read "Initialization finished"() -> (w1219:bool)
    n535 = case shown="True" w1219 {
      tunnel: [FALSE ("ShutDown") w1222] -> w1218
      frame False {
      }
      frame True {
        n536 = while {
          shift-right: [w1230] -> _
          shift-left: enum16{"Initialize", "Live", "Exit"}."Initialize" -> [w1231]
          shift-right: [w1228] -> _
          shift-left: errorcluster {"status"=FALSE, "code"=0, "source"=""} ("error in") -> [w1229]
          tunnel: [w1227] -> w1222
          shift-right: [w1225] -> _
          shift-left: TRUE -> [w1226]
          stop <- w1227 stop-if-true
          n537 = case shown="\"Live\"" w1231 {
            tunnel: [enum16{"Initialize", "Live", "Exit"}."Live" w1278 enum16{"Initialize", "Live", "Exit"}."Exit"] -> w1230
            tunnel: w1229 -> [w1237 w1277 w1351]
            tunnel: [w1234 w1276 w1350] -> w1228
            tunnel: [FALSE ("ShutDown") FALSE ("ShutDown") w1342] -> w1227
            tunnel: w1226 -> [w1232 w1273 w1341]
            tunnel: [w1232 w1272 w1341] -> w1225
            frame "Initialize", Default {
              n538 = flat-sequence {
                tunnel: [w1246] -> w1238
                tunnel: w1237 -> [w1246]
                tunnel: w1238 -> [w1260]
                tunnel: [w1259] -> w1236
                tunnel: w1236 -> [w1268]
                tunnel: [w1267] -> w1235
                tunnel: w1235 -> [w1271]
                tunnel: [w1271] -> w1234
                frame #0 {
                  n539 = local write "ShutDown"(cluster{"CoolOff":bool, "ShutDown":bool} {"CoolOff"=FALSE, "ShutDown"=FALSE} ("ShutDown")) -> ()
                  n540 = local write "SetStatus"(FALSE ("SetStatus")) -> ()
                  n541 = local write "GetStatus"(T18 {"GetDetector"=FALSE, "GetHardVer"=FALSE, "GetNVS"=FALSE, "GetVS"=FALSE, "GetSotfVer"=FALSE, "GetNHS"=FALSE, "GetHS"=FALSE} ("GetStatus")) -> ()
                  n542 = local write "SaveStatus"(FALSE ("Save")) -> ()
                  n543 = local write "CoolerON"(T17 {"SetTemp"=FALSE, "CoolerOn"=FALSE, "Stablized"=FALSE} ("CoolerON")) -> ()
                  n544 = local write "DevInit"(FALSE ("DevInit")) -> ()
                }
                frame #1 {
                  n545 = local read "TargetTemp"() -> (w1255:i32)
                  n546 = control-ref of="CurrentTemp"() -> (w1257:refnum<vi>)
                  n547 = control-ref of="GetStatus"() -> (w1258:refnum<vi>)
                  n548 = control-ref of="CoolerON"() -> (w1256:refnum<vi>)
                  n549 = call "AndorInit.vi"("TargetTemp"=w1255, "error in"=w1260, "CoolerONRef"=w1256, "GetStatusRef"=w1258, "CurrentTempRef"=w1257) -> ("GetStatus"=w1247:T18, "CurrentTemp"=w1254:i32, "CoolerON"=w1253:T17, "DevInit"=w1250:bool, "DevSize"=w1249:cluster{"xpixels":i32, "ypixels":i32}, "HardWVersion"=w1248:T14, "SoftWVersion"=w1251:T15, "Speeds"=w1252:T16, "error out"=w1259:errorcluster)  [unwired: 6 in]
                  n550 = local write "CurrentTemp"(w1254) -> ()
                  n551 = local write "SoftWVersion"(w1251) -> ()
                  n552 = local write "Speeds"(w1252) -> ()
                  n553 = local write "HardWVersion"(w1248) -> ()
                  n554 = local write "DevSize"(w1249) -> ()
                  n555 = local write "DevInit"(w1250) -> ()
                  n556 = local write "GetStatus"(w1247) -> ()
                  n557 = local write "CoolerON"(w1253) -> ()
                }
                frame #2 {
                  n558 = local read "MultiTrack"() -> (w1264:cluster{"StartRow":i32, "EndRow":i32})
                  n559 = local read "AcqSet"() -> (w1266:T11)
                  n560 = local read "Mode"() -> (w1265:T10)
                  n561 = call "AndorSet.vi"("error in"=w1268, "MultiTrack"=w1264, "AcqSet"=w1266, "Mode"=w1265) -> ("error out"=w1267:errorcluster, "SetStatus"=w1261:bool, "SetOut"=w1262:T13, "Timing"=w1263:T12)  [unwired: 4 in]
                  n562 = local write "SetOut"(w1262) -> ()
                  n563 = local write "Timing"(w1263) -> ()
                  n564 = local write "SetStatus"(w1261) -> ()
                }
                frame #3 {
                  n565 = call "Display Message to User2"("Enable"=TRUE, "Message"="Andor now is ready!!!") -> ()  [unwired: 8 in, 2 out]
                }
              }
            }
            frame "Live" {
              n566 = event shown="[2] \"Galvo Stop\": Value Change" {
                selector: _ -> [_ _ _ _ _ _]
                dyn-events: _ -> [_ _ _ _ _ _]
                timeout: 0 -> [_ _ _ _ _ _]
                tunnel: [enum16{"Initialize", "Live", "Exit"}."Live" enum16{"Initialize", "Live", "Exit"}."Live" enum16{"Initialize", "Live", "Exit"}."Live" enum16{"Initialize", "Live", "Exit"}."Live" enum16{"Initialize", "Live", "Exit"}."Live" enum16{"Initialize", "Live", "Exit"}."Exit"] -> w1278
                tunnel: w1277 -> [w1281 w1290 w1297 w1309 w1314 w1339]
                tunnel: [w1280 w1290 w1297 w1308 w1312 w1339] -> w1276
                tunnel: w1273 -> [w1279 w1288 w1295 w1301 w1311 w1338]
                tunnel: [w1279 w1287 w1294 w1301 w1311 w1338] -> w1272
                event Timeout {
                  n567 = event-data() -> ()  [unwired: 1 in, 3 out]
                  n568 = Wait Until Next ms Multiple(millisecond multiple=u32 500) -> ()  [unwired: 1 out]
                  n569 = case shown="True" w1279 {
                    tunnel: w1281 -> [w1284 w1285]
                    tunnel: [w1284 w1285] -> w1280
                    frame False {
                    }
                    frame True {
                      n570 = call <userlib>:"GetTemperature.vi"("error in (no error)"=w1285) -> ("temperature"=w1286:i32)  [unwired: 3 in, 3 out]
                      n571 = local write "CurrentTemp"(w1286) -> ()
                    }
                  }
                }
                event "Galvo Scan": Value Change {
                  n572 = event-data() -> ()  [unwired: 1 in, 6 out]
                  n573 = case shown="False" w1288 {
                    tunnel: w1288 -> [w1291 w1293]
                    tunnel: [w1291 w1292] -> w1287
                    frame False {
                    }
                    frame True {
                      n574 = Not(x=w1293) -> (.not. x?=w1292:bool)
                    }
                  }
                }
                event "Galvo Stop": Value Change {
                  n575 = event-data() -> ()  [unwired: 1 in, 6 out]
                  n576 = case shown="False" w1295 {
                    tunnel: w1295 -> [w1299 w1300]
                    tunnel: [w1298 w1300] -> w1294
                    frame False {
                      n577 = Not(x=w1299) -> (.not. x?=w1298:bool)
                    }
                    frame True {
                    }
                  }
                }
                event "Set": Value Change {
                  n578 = event-data() -> ()  [unwired: 1 in, 6 out]
                  n579 = local read "AcqSet"() -> (w1306:T11)
                  n580 = local read "MultiTrack"() -> (w1305:cluster{"StartRow":i32, "EndRow":i32})
                  n581 = local read "Mode"() -> (w1307:T10)
                  n582 = call "AndorSet.vi"("error in"=w1309, "MultiTrack"=w1305, "AcqSet"=w1306, "Mode"=w1307) -> ("error out"=w1308:errorcluster, "SetStatus"=w1303:bool, "SetOut"=w1302:T13, "Timing"=w1304:T12)  [unwired: 4 in]
                  n583 = local write "Timing"(w1304) -> ()
                  n584 = local write "SetStatus"(w1303) -> ()
                  n585 = local write "SetOut"(w1302) -> ()
                }
                event "AndorSnap": Value Change {
                  n586 = event-data() -> ()  [unwired: 1 in, 6 out]
                  n587 = flat-sequence {
                    tunnel: [w1317] -> w1315
                    tunnel: w1314 -> [w1320]
                    tunnel: w1315 -> [w1332]
                    tunnel: [TRUE ("SaveStatus")] -> w1313
                    tunnel: [w1329] -> w1312
                    frame #0 {
                      n588 = case shown="No Error" w1320 {
                        tunnel: w1320 -> [w1323 w1328]
                        tunnel: [w1322 FALSE ("SaveStatus")] -> w1319
                        tunnel: [w1321 w1328] -> w1317
                        frame No Error {
                          n589 = local read "AcqSet"() -> (w1325:T11)
                          n590 = Unbundle By Name(w1325) -> ("KineticNum"=w1324:i32)
                          n591 = call "AndorSaveasSif.vi"("error in"=w1323, "KinNumber"=w1324, "FilePath"="FilePath") -> ("error out"=w1321:errorcluster, "SaveStatus"=w1322:bool)  [unwired: 7 in]
                        }
                        frame Error {
                        }
                      }
                      n592 = Not(x=w1319) -> (.not. x?=→"SaveStatus":bool)
                    }
                    frame #1 {
                      n593 = call <userlib>:"StartAcquisition.vi"("error in (no error)"=w1332) -> ("error out"=w1331:errorcluster)  [unwired: 1 in, 1 out]
                      n594 = while {
                        tunnel: w1331 -> [w1337]
                        tunnel: [w1334] -> w1329
                        stop <- w1333 continue-if-true
                        n595 = call <userlib>:"GetStatus.vi"("error in (no error)"=w1337) -> ("error out"=w1334:errorcluster, "status"=w1336:T30)  [unwired: 2 in, 1 out]
                        n596 = Equal?(x=w1336, y=Error_Code_Enum_typedef."DRV_ACQUIRING") -> (x = y?=w1333:bool)
                      }
                    }
                  }
                  n597 = local write "SaveStatus"(w1313) -> ()
                }
                event "Exit": Value Change {
                  n598 = event-data() -> ()  [unwired: 1 in, 6 out]
                }
              }
            }
            frame "Exit" {
              n599 = local read "CoolerON"() -> (w1349:T17)
              n600 = Unbundle By Name(w1349) -> ("SetTemp"=w1348:bool, "CoolerOn"=w1347:bool)
              n601 = control-ref of="CurrentTemp"() -> (w1346:refnum<vi>)
              n602 = control-ref of="ShutDown"() -> (w1344:refnum<vi>)
              n603 = call "AndorShutdown.vi"("ShutDownRef"=w1344, "CurrentTempRef"=w1346, "error in"=w1351, "CoolerON"=w1347, "SetTemp"=w1348) -> ("error out"=w1350:errorcluster, "ShutDown"=w1343:cluster{"CoolOff":bool, "ShutDown":bool}, "CurrentTemp"=w1345:i32)  [unwired: 4 in]
              "ShutDown" <- w1343
              n604 = local write "CurrentTemp"(w1345) -> ()
              n605 = Unbundle By Name(w1343) -> ("ShutDown"=w1342:bool)  [unwired: 1 out]
            }
          }
        }
      }
    }
  }
